vi "Lockin_time.vi"(8 "error in (no error)":errorcluster, 11 "Transport":refnum<class "Transport.lvclass">) -> (0 "error out":errorcluster, 3 "Transport out":refnum<class "Transport.lvclass">)   [LabVIEW 2019, in "Transport.lvclass"]
uses:
  Transport.lvclass
  Control Experiment/Control Experiment.lvclass
  <userlib>/LevyLab/Lockin-Multichannel/Instrument.Lockin/Instrument.Lockin.lvclass
  <userlib>/LevyLab/Lockin-Multichannel/Instrument.Lockin/Typedefs/Results Type--Enum.ctl
  <vilib>/PRIrvin/XY Utilities/xy_utilities.lvlib
  <vilib>/PRIrvin/XY Utilities/subVIs/Divide float (multiple).vi
  <vilib>/PRIrvin/XY Utilities/subVIs/Multiply float (multiple).vi
  8746f36a-7fba-47b8-9d0d-e5093f5f71bf.vi
  f6961605-28f7-45ab-8853-bc719731420b.vi
  <vilib>/PRIrvin/XY Utilities/subVIs/Get X and Y (single).vi
  <userlib>/LevyLab/Instrument Framework/Instrument Types/Cryostat/Typedefs/Magnet Mode--Enum.ctl
  <userlib>/LevyLab/Instrument Framework/Instrument Types/Cryostat/Instrument.Cryostat.lvclass
  <vilib>/Utility/Data Type/NI_Data Type.lvlib
  C:/Program Files/National Instruments/LabVIEW 2019/vi.lib/JKI/JKI SMO/SMO/SMO.lvclass
  <userlib>/LevyLab/Instrument Framework/Instrument Types/Lockin/Instrument.LockinAPI.lvclass
  <userlib>/LevyLab/Instrument Framework/Instrument Types/Amplifier/Instrument.Amplifier.lvclass
  <userlib>/LevyLab/Instrument Framework/Instrument Types/CBridge/Instrument.CBridge.lvclass
  <userlib>/LevyLab/Instrument Framework/Instrument Types/Delay Line/Instrument.DelayLine.lvclass
  <userlib>/LevyLab/Instrument Framework/Instrument Types/Strain/Instrument.Strain.lvclass
  <userlib>/LevyLab/Instrument Framework/Instrument Types/VNA/Instrument.VNA.lvclass
  <userlib>/LevyLab/Instrument Framework/Instrument Types/VSource/Instrument.VSource.lvclass
  Control Experiment/Typedefs/Instrument Types--enum.ctl
  <userlib>/LevyLab/Instrument Framework/Instrument/Instrument.lvclass
  Attributes/Instrument Attributes.lvlib
  <vilib>/PRIrvin/XY Utilities/subVIs/Get X and Y (multiple).vi
  <userlib>/LevyLab/Debug/Debug.lvlib
  28257cb1-27ee-4ed9-8846-d02f057abbea.vi
  C:/Program Files/National Instruments/LabVIEW 2019/user.lib/LevyLab/Instrument Framework/Instrument Types/Lockin/Instrument.LockinAPI.lvclass
  <userlib>/LevyLab/Instrument Framework/Instrument Types/Cryostat/Typedefs/Magnet Axis--Enum.ctl
panel:
  in  "Stop":bool
  in  "Tab Control":T1(tab)
  in  "Hold?":bool
  out "Instrument Status":string
  out "Mean":dbl[](array[numeric]) format="%#_6p"
  in  "refresh (ms)":u32=1000
  out "Experiment Description":string="this is the experiment description"
  out "Experiment Folder":string="1 -  Folder Name"
  out "X Channels":dbl[](array[numeric]) format="%#_6p"
  out "Y Channels":dbl[](array[numeric]) format="%#_6p"
  out "State History":string
  in  "T_hold (K)":dbl=1000.0
  out "Y":cluster{"Wavenumber":dbl[], "Data":dbl[]}[](graph)
  out "X":cluster{"Y":dbl[], "Y":dbl[]}[](graph)
  out "Mean":cluster{"Wavenumber":dbl[], "Data":dbl[]}[](graph)
  out "X (2)":cluster{"Y":dbl[], "Y":dbl[]}[](graph)
  in  "Units":enum16{"ohms & siemens", "h/e2 & e2/h"}(ring)
  out "G vs time":cluster{"Wavenumber":dbl[], "Data":dbl[]}[](graph)
  out "R vs time":cluster{"Wavenumber":dbl[], "Data":dbl[]}[](graph)
  in  "Electrodes":T2(array[cluster])
  out "T vs time":cluster{"X-array":dbl[], "Y-array":dbl[]}[](graph)
  out "R vs T":cluster{"Wavenumber":dbl[], "Data":dbl[]}[](graph)
  out "B vs time":cluster{"X-array":dbl[], "Y-array":dbl[]}[](graph)
  out "R vs B":cluster{"Wavenumber":dbl[], "Data":dbl[]}[](graph)
  in  "Axis":T3
  out "Angle vs time":cluster{"X-array":dbl[], "Y-array":dbl[]}[](graph)
  out "R vs Angle":cluster{"Wavenumber":dbl[], "Data":dbl[]}[](graph)
  # "Measurements"
  # "Configuration"
  # "Status"
  # "Metadata*"
  # "VI Description"
  # "Record the lockin outputs, along with the other configured instruments, as a function of time. On each refresh interval it reads every instrument and records one point. It runs until stopped. The refresh time can be changed while the VI is running (setRefreshTime)."
  # "*Change these values in Transport Server"
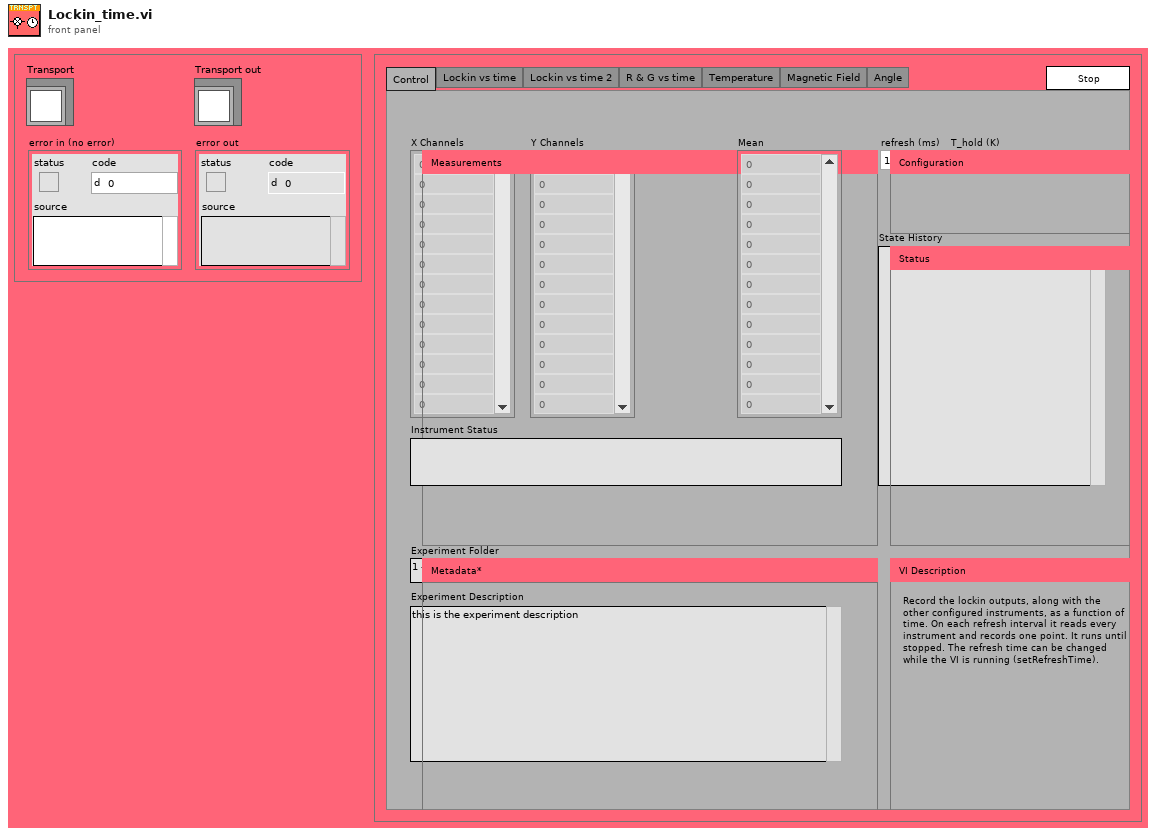
[diagram p1: front panel]
types:
  T1 = enum32{"Control", "Lockin vs time", "Lockin vs time 2", "R & G vs time", "Temperature", "Magnetic Field", "Angle"}
  T2 = cluster{"I+":i32, "I-":i32, "V+":i32, "V-":i32}[]
  T3 = typedef "Instrument.Cryostat.lvclass/Magnet Axis--Enum.ctl" = enum16{"X", "Y", "Z"}
  T4 = enum32{"Invalid", "Standard", "Closed", "Hidden", "Minimized", "Maximized"}
  T5 = enum32{"invalid app kind", "Development System", "Run Time System", "Student Edition", "Embedded LabVIEW", "Evaluation", "Custom"}
  T6 = typedef "Control Experiment.lvclass/Instrument Types--enum.ctl" = enum16{"DAQ", "Amplifier", "Temperature", "Magnet", "Rotator", "Level", "Capacitance", "Delay Line", "Strain Cell", "VNA", "Source"}
  T7 = typedef "Instrument.Cryostat.lvclass/Magnet Mode--Enum.ctl" = enum16{"Persistent", "Driven"}
  T8 = typedef "Instrument.Lockin.lvlib/Instrument.Lockin.lvclass/Results Type--Enum.ctl" = enum16{"X", "Y", "R", "Theta", "Mean"}
  T9 = typedef "Control Experiment.lvclass/Instrument Classes--cluster.ctl" = cluster{"DAQ":refnum<class "Instrument.LockinAPI.lvclass">, "Amplifier":refnum<class "Instrument.Amplifier.lvclass">, "Temperature":refnum<class "Instrument.Cryostat.lvclass">, "Magnet":refnum<class "Instrument.Cryostat.lvclass">, "Rotator":refnum<class "Instrument.Cryostat.lvclass">, "Level":refnum<class "Instrument.Cryostat.lvclass">, "Capacitance":refnum<class "Instrument.CBridge.lvclass">, "Delay Line":refnum<class "Instrument.DelayLine.lvclass">, "Strain Cell":refnum<class "Instrument.Strain.lvclass">, "VNA":refnum<class "Instrument.VNA.lvclass">, "Source":refnum<class "Instrument.VSource.lvclass">}
  T10 = cluster{"Core":cluster{"Current VI Reference":refnum<vi>, "Close Panel on Exit?":bool}, "Transport":refnum<class "Transport.lvclass">, "C.E.":refnum<class "Control Experiment.lvclass">, "Instruments":T9, "path":path, "time":dbl, "temperature":dbl, "magnet field":dbl, "magnet rate":dbl, "magnet hold":dbl, "magnet rate hold":dbl, "angle":dbl, "Lockin X":dbl[], "Lockin Y":dbl[], "Lockin Mean":dbl[], "Excitation":dbl[], "AO":dbl[], "AI":dbl[], "R2T":dbl[], "R4T":dbl[], "G2T":dbl[], "G4T":dbl[], "Execution:State":enum32{"Bad", "Idle", "Run top level", "Running"}}
  T11 = enum32{"Bad", "Idle", "Run top level", "Running"}
  T12 = cluster{"Current VI Reference":refnum<vi>, "Close Panel on Exit?":bool}
  T13 = cluster{"I-":i32, "I+":i32, "V1-":i32, "V1+":i32, "I2-":i32, "I2+":i32, "V2-":i32, "V2+":i32}
  T14 = typedef "LV-Data.lvclass/Dictionary--cluster.ctl" = cluster{"key":string, "value":variant}
  T15 = typedef "Instrument.Lockin.lvlib/Instrument.DAQ.lvclass/AO.Channel--Cluster--Array.ctl" = T16[]
  T16 = typedef "Instrument.Lockin.lvlib/Instrument.DAQ.lvclass/AO.Channel--Cluster.ctl" = cluster{"Enable?":bool, "Channel":i32, "Amplitude":dbl, "Offset":dbl, "Frequency":dbl, "Phase":dbl, "Function":T17, "Sweeping?":bool, "Limit AC":bool, "Limit DC?":bool, "Duty Cycle":bool}
  T17 = typedef "Instrument.Lockin.lvlib/Instrument.DAQ.lvclass/AO.Channel.Function--Enum.ctl" = enum16{"sine", "square", "triangle", "saw"}
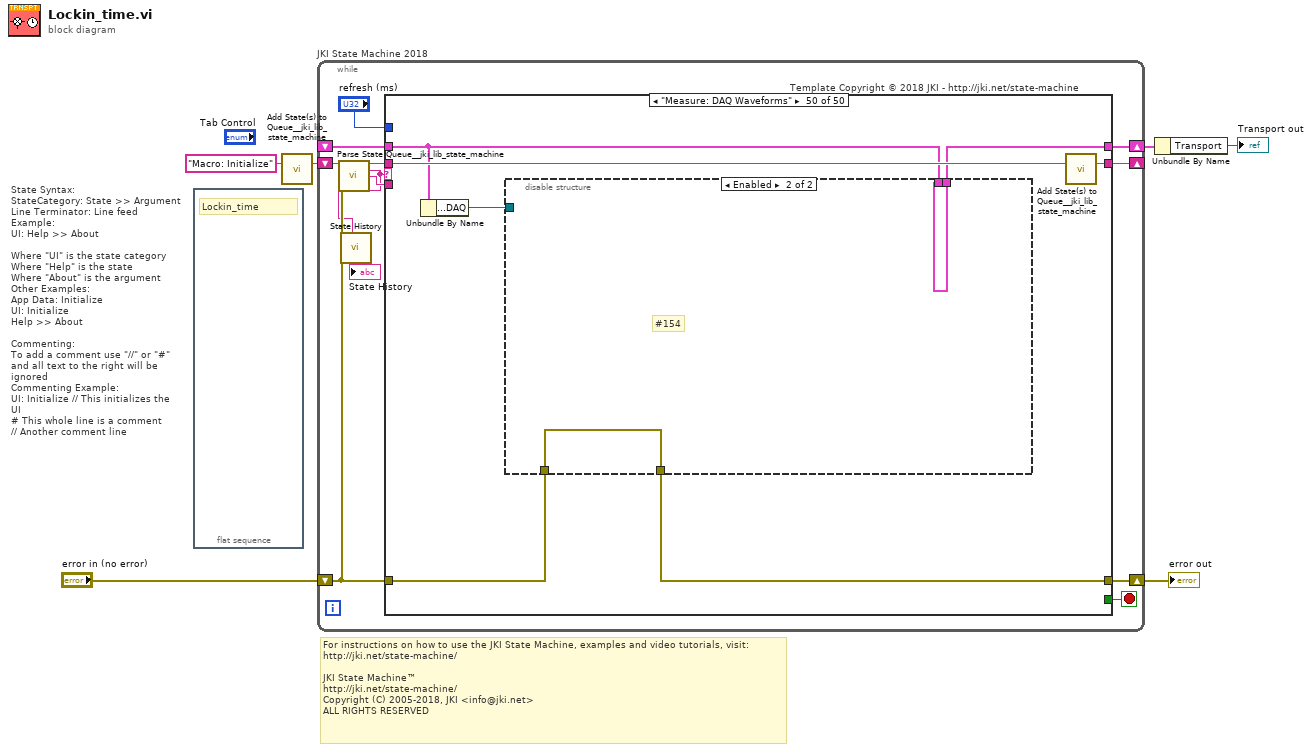
[diagram p0: block diagram]
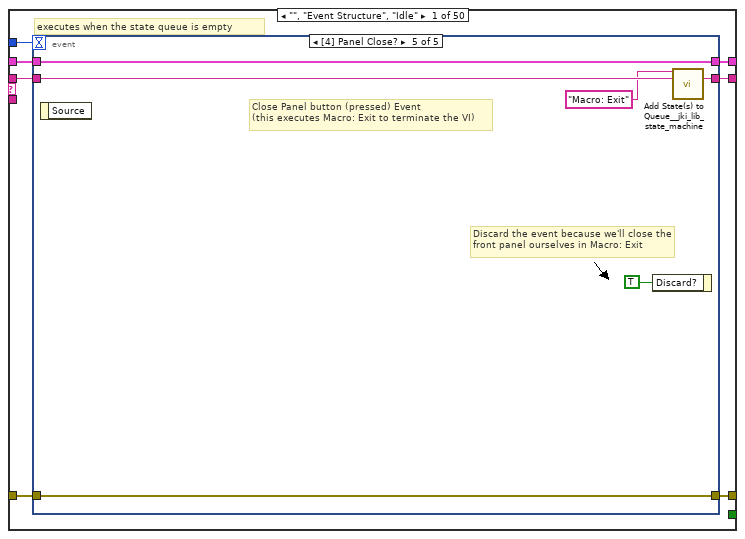
[diagram p2: hidden frame]
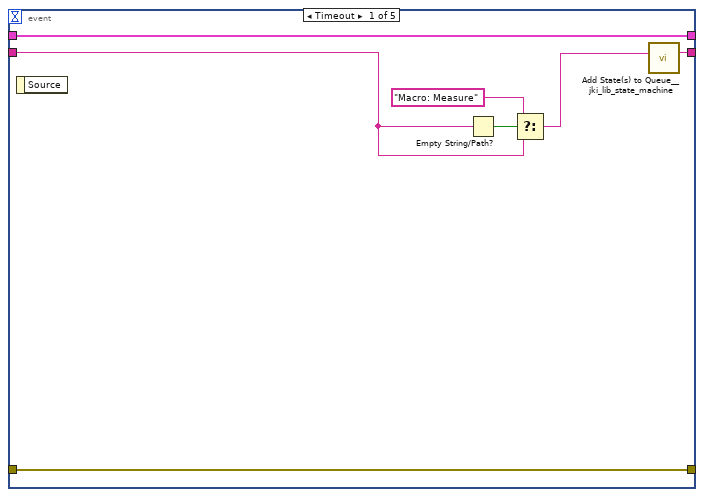
[diagram p3: hidden frame]
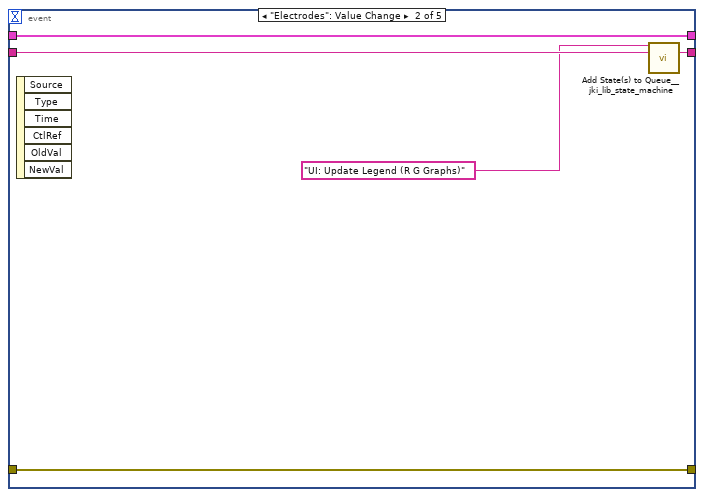
[diagram p4: hidden frame]
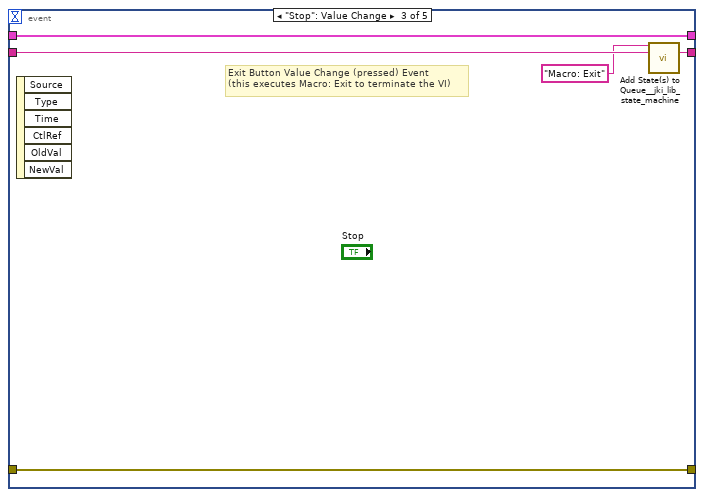
[diagram p5: hidden frame]
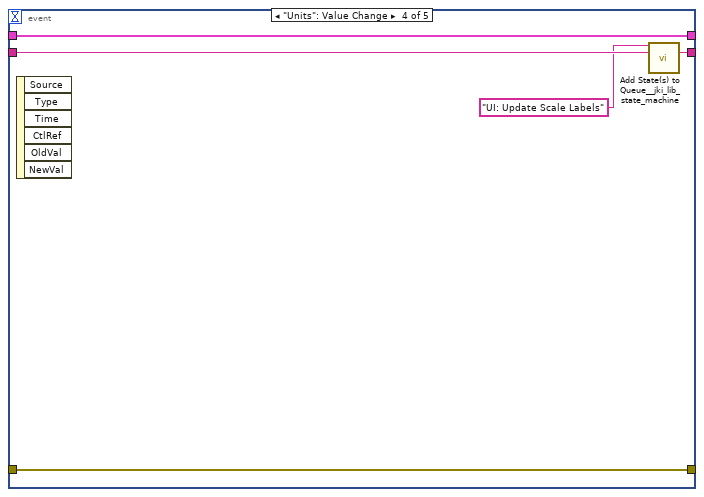
[diagram p6: hidden frame]
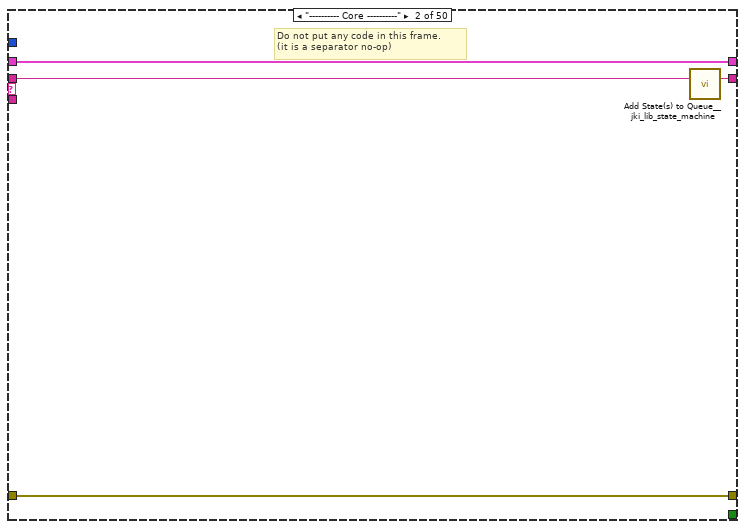
[diagram p7: hidden frame]
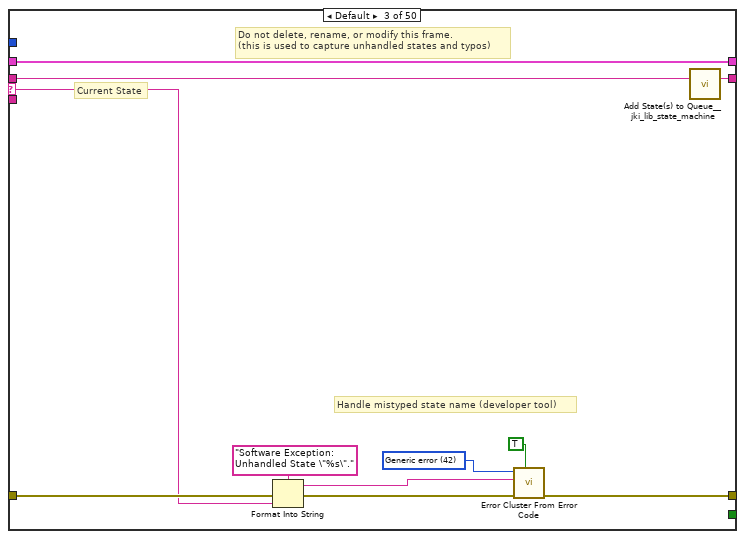
[diagram p8: hidden frame]
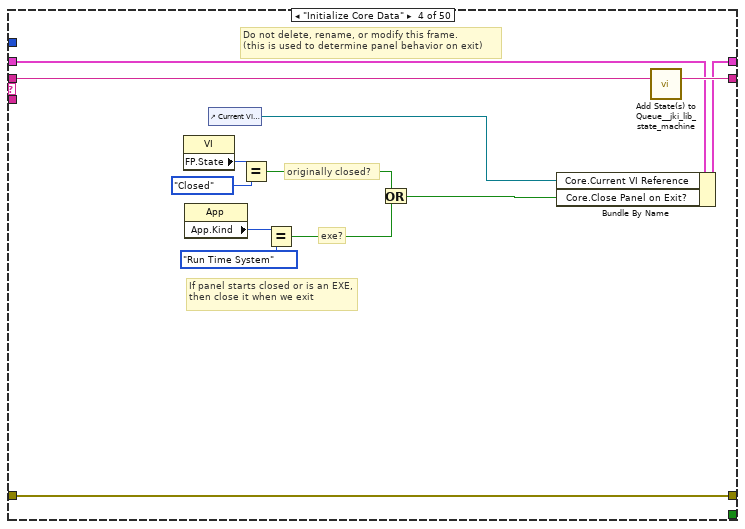
[diagram p9: hidden frame]
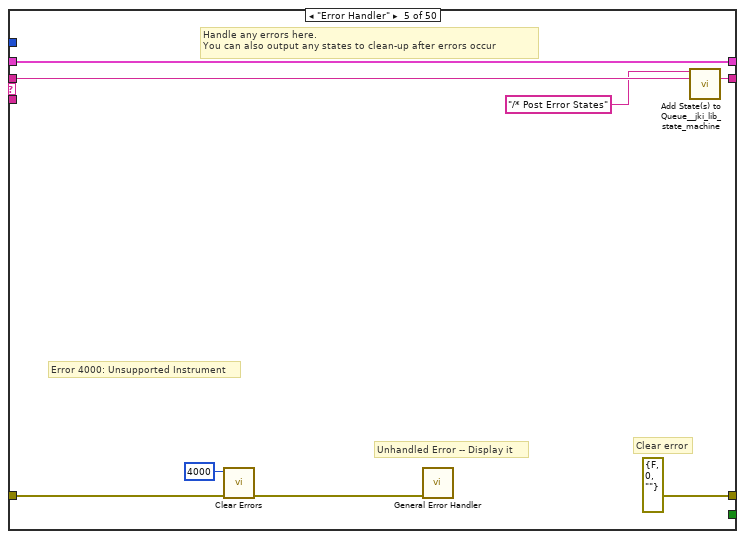
[diagram p10: hidden frame]
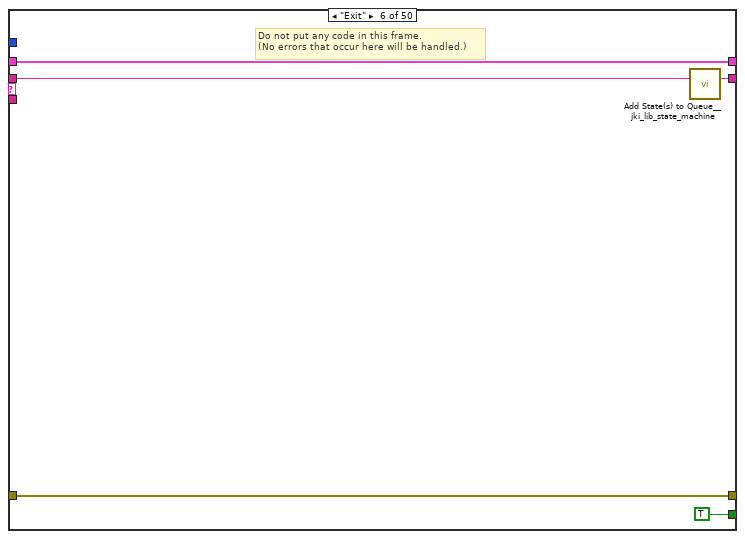
[diagram p11: hidden frame]
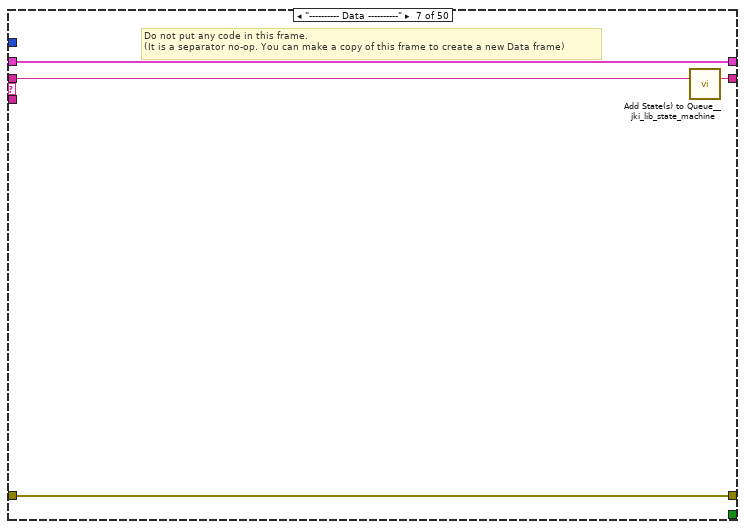
[diagram p12: hidden frame]
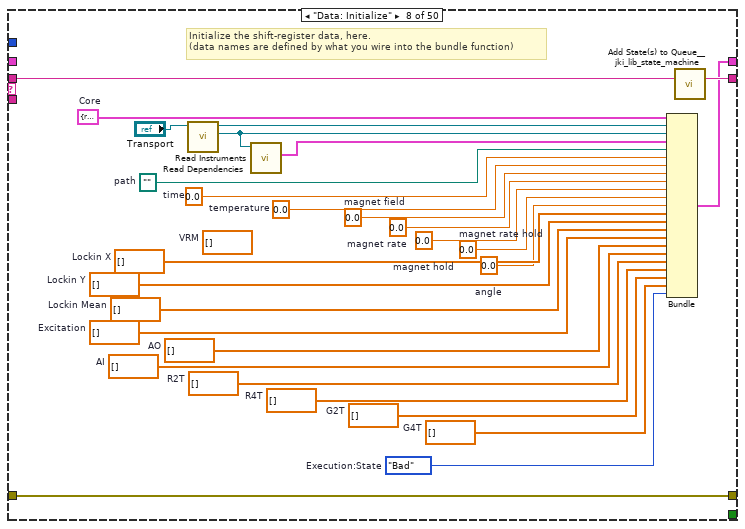
[diagram p13: hidden frame]
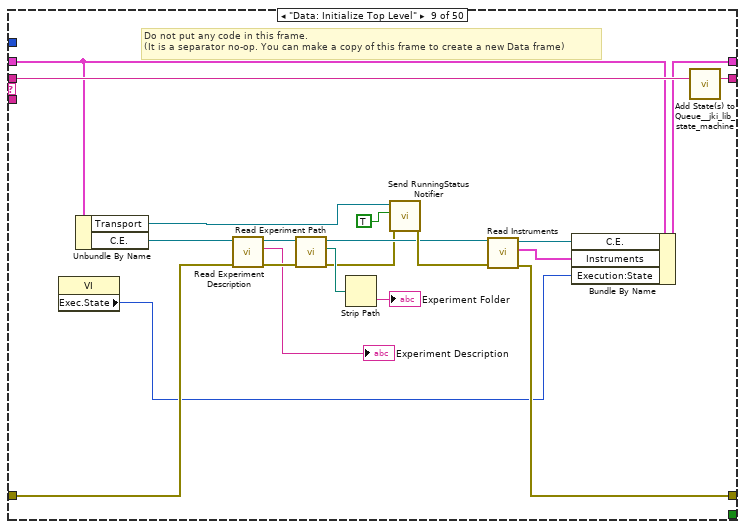
[diagram p14: hidden frame]
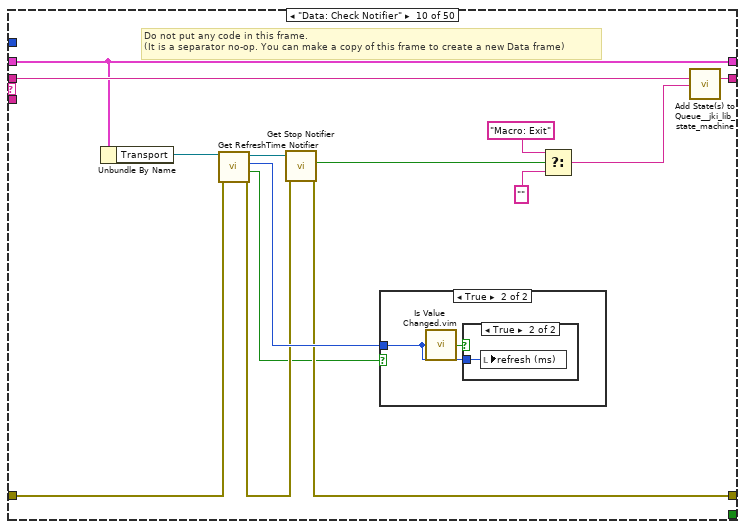
[diagram p15: hidden frame]
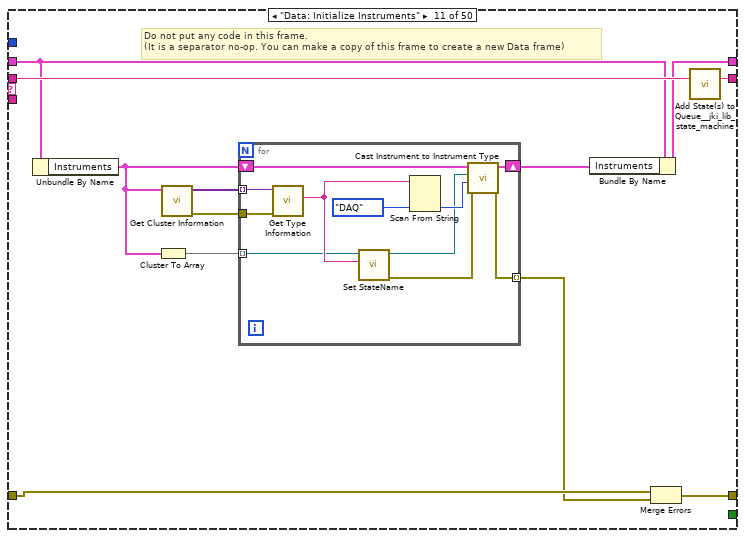
[diagram p18: hidden frame]
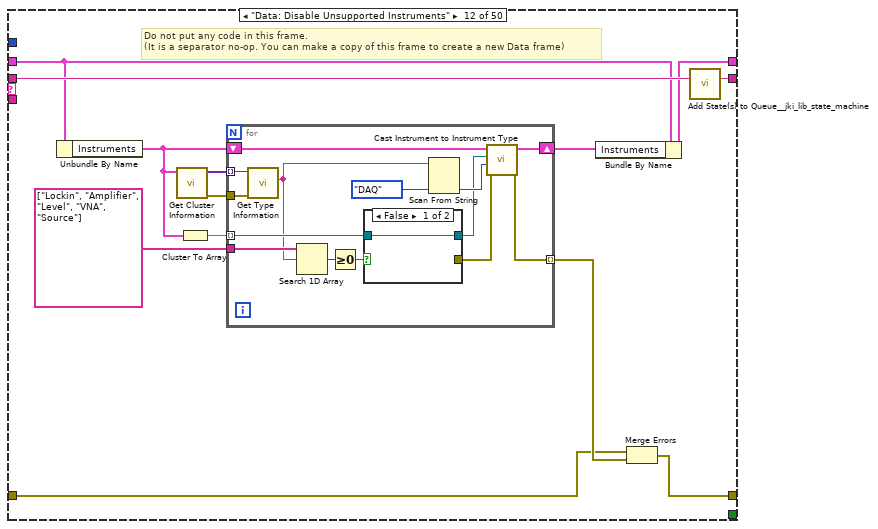
[diagram p19: hidden frame]
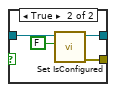
[diagram p20: hidden frame]
diagram:
  # "For instructions on how to use the JKI State Machine, examples and video tutorials, visit:\nhttp://jki.net/state-machine/\n\nJKI State Machine™\nhttp://jki.net/state-machine/\nCopyright (C) 2005-2018, JKI <info@jki.net>\nALL RIGHTS RESERVED"
  # "State Syntax:\nStateCategory: State >> Argument\nLine Terminator: Line feed\nExample:\nUI: Help >> About\n\nWhere \"UI\" is the state category\nWhere \"Help\" is the state\nWhere \"About\" is the argument\nOther Examples:\nApp Data: Initialize\nUI: Initialize\nHelp >> About\n\nCommenting:\nTo add a comment use \"//\" or \"#\" and all text to the right will be ignored\nCommenting Example:\nUI: Initialize // This initializes the UI\n# This whole line is a comment\n// Another comment line"
  n1 = flat-sequence {
    frame #0 {
      # "Lockin_time"
    }
  }
  n2 = call <vilib>:"Add State(s) to Queue__jki_lib_state_machine.vi"("State(s) in (\"\")"="Macro: Initialize") -> ("States Out"=w6:string)  [unwired: 14 in]
  n3 = while "JKI State Machine 2018" {
    shift-right: [w12] -> w2
    shift-left: _ -> [w11]
    shift-right: [w15] -> w3
    shift-left: "error in (no error)" -> [w10]
    shift-right: [w14] -> _
    shift-left: w6 -> [w16]
    stop <- w13 stop-if-true
    # "Template Copyright © 2018 JKI - http://jki.net/state-machine"
    n4 = call <vilib>:"Parse State Queue__jki_lib_state_machine.vi"("State Queue"=w16, "Error In (no error)"=w10) -> ("Remaining States"=w18:string, "Current State"=w8:string, "Arguments"=w17:string)  [unwired: 11 in]
    n5 = call <userlib>:"State History.vi"("Current State"=w8) -> ("History"=→"State History":string)  [unwired: 9 in, 1 out]
    n6 = case shown="\"Measure: DAQ Waveforms\"" w8 {
      selector: w8 -> [_ _ w58 _ _ _ _ _ _ _ _ _ _ _ _ _ _ _ _ _ _ _ _ _ _ _ _ _ _ _ _ _ _ _ _ _ _ _ _ _ _ _ _ _ _ _ _ _ _ _]
      tunnel: w18 -> [w25 w57 w62 w81 w89 w94 w98 w126 w146 w160 w175 w199 w230 w266 w278 w327 w348 w360 w366 w378 w413 w447 w466 w472 w483 w599 w630 w634 w639 w644 w649 w660 w673 w684 w688 w710 w725 w738 w749 w768 w802 w833 w845 w866 w899 w921 w943 w965 w999 w1009]
      tunnel: w17 -> [_ _ _ _ _ _ _ _ _ _ _ _ _ _ _ _ _ _ _ _ _ _ w452 w467 w477 w596 w624 _ _ _ _ _ _ _ _ w690 _ _ _ _ _ _ _ _ _ _ _ _ _ _]
      tunnel: w11 -> [w23 w54 w60 w74 w86 w92 w95 _ w142 w156 w172 w196 w227 w261 w275 w311 w345 w357 w363 w375 w410 w444 w463 w470 w479 w593 w627 w631 w636 w640 w646 w657 w670 w681 w685 w708 w716 w735 w742 w762 w795 w831 w843 w864 w889 w911 w933 w955 w996 w1006]
      tunnel: [w22 w55 w64 w78 errorcluster {"status"=FALSE, "code"=0, "source"=""} ("error out") w91 w96 w123 w137 w150 w171 w187 w226 w253 w274 w318 w343 w358 w362 w374 w405 w445 w464 w468 w480 w597 w628 w632 w637 w642 w647 w652 w671 w682 w686 w694 w718 w736 w740 w756 w790 w823 w839 w862 w887 w909 w931 w953 w980 w1004] -> w15
      tunnel: w10 -> [w21 w55 w63 w78 w82 w91 w96 w123 w141 w149 w165 w189 w225 w259 w273 w317 w341 w358 w364 w376 w411 w445 w464 w469 w481 w597 w628 w632 w637 w642 w647 w651 w671 w682 w686 w693 w720 w736 w739 w760 w793 w819 w836 w852 w891 w913 w935 w957 w973 w1003]
      tunnel: [w24 w56 w61 w80 w88 w93 w97 w125 w145 w159 w174 w198 w229 w265 w277 w326 w347 w359 w365 w377 w412 w446 w465 w471 w482 w598 w629 w633 w638 w643 w648 w659 w672 w683 w687 w709 w724 w737 w748 w767 w801 w832 w844 w865 w898 w920 w942 w964 w998 w1008] -> w14
      tunnel: [_ _ _ _ _ TRUE _ _ _ _ _ _ _ _ _ _ _ _ _ _ _ _ _ _ _ _ _ _ _ _ _ _ _ _ _ _ _ _ _ _ _ _ _ _ _ _ _ _ _ _] -> w13
      tunnel: [w20 w54 w60 w79 w86 w92 w95 w124 w143 w156 w173 w197 w228 w260 w276 w312 w344 w357 w363 w375 w410 w444 w463 w470 w479 w593 w627 w631 w636 w640 w646 w657 w670 w681 w685 w707 w717 w735 w741 w761 w794 w830 w842 w863 w890 w912 w934 w956 w997 w1007] -> w12
      tunnel: "refresh (ms)" -> [w19 _ _ _ _ _ _ _ _ _ _ _ _ _ _ _ _ _ _ _ _ _ _ _ _ _ _ _ _ _ _ _ _ _ _ _ _ _ _ _ _ _ _ _ _ _ _ _ _ _]
      frame "", "Event Structure", "Idle" {
        # "executes when the state queue is empty"
        n7 = event shown="[4] Panel Close?" {
          selector: _ -> [_ _ _ _ _]
          dyn-events: _ -> [_ _ _ _ _]
          timeout: w19 -> [_ _ _ _ _]
          tunnel: w25 -> [w28 w37 w42 w47 w53]
          tunnel: [w32 w36 w41 w46 w52] -> w24
          tunnel: w23 -> [w30 w34 w39 w44 w50]
          tunnel: [w31 w35 w40 w45 w51] -> w22
          tunnel: w21 -> [w31 w35 w40 w45 w51]
          tunnel: [w30 w34 w39 w44 w50] -> w20
          event Timeout {
            n8 = event-data() -> ()  [unwired: 1 in, 1 out]
            n9 = Empty String/Path?(string/path=w28) -> (empty?=w29:bool)
            n10 = Select(t="Macro: Measure" ("State(s) in Front (\"\")"), s=w29, f=w28) -> (s? t:f=w26:string)
            n11 = call <vilib>:"Add State(s) to Queue__jki_lib_state_machine.vi"("State(s) in (\"\")"=w26) -> ("States Out"=w32:string)  [unwired: 14 in]
          }
          event "Electrodes": Value Change {
            n12 = event-data() -> ()  [unwired: 1 in, 6 out]
            n13 = call <vilib>:"Add State(s) to Queue__jki_lib_state_machine.vi"("State(s) in Front (\"\")"="UI: Update Legend (R G Graphs)" ("State(s) in Front (\"\")"), "State(s) in (\"\")"=w37) -> ("States Out"=w36:string)  [unwired: 13 in]
          }
          event "Stop": Value Change {
            # "Exit Button Value Change (pressed) Event\n(this executes Macro: Exit to terminate the VI)"
            n14 = event-data() -> ()  [unwired: 1 in, 6 out]
            n15 = call <vilib>:"Add State(s) to Queue__jki_lib_state_machine.vi"("State(s) in Front (\"\")"="Macro: Exit", "State(s) in (\"\")"=w42) -> ("States Out"=w41:string)  [unwired: 13 in]
          }
          event "Units": Value Change {
            n16 = event-data() -> ()  [unwired: 1 in, 6 out]
            n17 = call <vilib>:"Add State(s) to Queue__jki_lib_state_machine.vi"("State(s) in Front (\"\")"="UI: Update Scale Labels", "State(s) in (\"\")"=w47) -> ("States Out"=w46:string)  [unwired: 13 in]
          }
          event Panel Close? {
            # "Discard the event because we'll close the front panel ourselves in Macro: Exit"
            # "Close Panel button (pressed) Event\n(this executes Macro: Exit to terminate the VI)"
            n18 = event-data() -> ()  [unwired: 1 in, 1 out]
            n19 = event-data("Discard?"=TRUE) -> ()  [unwired: 1 in, 1 out]
            n20 = call <vilib>:"Add State(s) to Queue__jki_lib_state_machine.vi"("State(s) in Front (\"\")"="Macro: Exit", "State(s) in (\"\")"=w53) -> ("States Out"=w52:string)  [unwired: 13 in]
          }
        }
      }
      frame "---------- Core ----------" {
        # "Do not put any code in this frame.\n(it is a separator no-op)"
        n21 = call <vilib>:"Add State(s) to Queue__jki_lib_state_machine.vi"("State(s) in (\"\")"=w57) -> ("States Out"=w56:string)  [unwired: 14 in]
      }
      frame Default {
        w67 = 42 items=["No error", "Argument error", "Memory is full", "Out of zone", "End of file", "File already open", "Generic file I/O error", "File not found", "File permission error", "Disk is full", "Duplicate path", "Too many files open", "System feature not enabled", "Resource file not found", "Cannot add resource", "Resource not found", "Image not found", "Image memory error", "Pen does not exist", "Config type invalid", "Config token not found", "Config parse error", "Config memory error", "Bad external code format", "Bad external code offset", "External code not present", "Null window", "Destroy window error", "Null menu", "Print aborted", "Bad print record", "Print driver error", "Windows error during printing", "Memory error during printing", "Print dialog error", "Generic print error", "Invalid device refnum", "Device not found", "Device parameter error", "Device unit error", "Cannot open device", "Device call aborted", "Generic error", "Cancelled by user", "Object ID too low", "Object ID too high", "Object not in heap", "Unknown heap", "Unknown object (invalid DefProc)", "Unknown object (DefProc not in table)", "Message out of range", "Invalid (null) method", "Unknown message", "Manager call not supported", "Bad address", "Network operation in progress", "Network operation timed out", "Connection is busy", "Network attribute not supported", "Network error", "Address in use", "System out of memory", "Connection aborted", "Connection refused", "Not connected", "Already connected", "Connection closed", "Initialization error (interapplication manager)", "Bad occurrence", "Wait on unbound occurrence handler", "Occurrence queue overflow", "Datalog type conflict", "Unused", "Unrecognized type (interapplication manager)", "Memory corrupt", "Failed to make temporary DLL", "Old CIN version", "Drag socket not found", "Failed to load drop-object", "Failed to register OLE object", "Failed to release OLE object", "Format specifier type mismatch", "Unknown format specifier", "Too few format specifiers", "Too many format specifiers", "Scan failed", "Newer CIN version", "Error converting to variant", "Runtime menu error", "Password tampered", "Variant attribute not found", "Incompatible variant data type", "Event data is not available", "Event Store is not present", "Occurrence is not found", "Event Queue is not created", "Event info is not available", "Refnum passed is NULL", "Error retrieving Class GUID", "Error retrieving CoClass GUID", "Error retrieving TypeLib GUID.", "Bad built application magic bytes.", "Specific driver is different from the specific driver associated with the Logical Name.", "There is no session opened to the class driver.", "Max Error", "MAX - Error with config objects", "MAX - Error loading configuration", "MAX - Group not supported"]
        # "Current State"
        # "Do not delete, rename, or modify this frame.\n(this is used to capture unhandled states and typos)"
        # "Handle mistyped state name (developer tool)"
        n22 = Format Into String(format string="Software Exception: Unhandled State \"%s\"." ("message"), error in=w63, w58) -> (resulting string=w66:string, error out=w65:errorcluster)  [unwired: 1 in]
        n23 = call <vilib>:"Error Cluster From Error Code.vi"("show call chain? (False)"=TRUE, "error in (no error)"=w65, "error message (\"\")"=w66, "error code (0)"=w67) -> ("error out"=w64:errorcluster)  [unwired: 5 in]
        n24 = call <vilib>:"Add State(s) to Queue__jki_lib_state_machine.vi"("State(s) in (\"\")"=w62) -> ("States Out"=w61:string)  [unwired: 14 in]
      }
      frame "Initialize Core Data" {
        # "Do not delete, rename, or modify this frame.\n(this is used to determine panel behavior on exit)"
        # "originally closed?"
        # "exe?"
        # "If panel starts closed or is an EXE, then close it when we exit"
        n25 = property class="VI"() -> ("FP.State"=w71:T4)  [unwired: 2 in, 2 out]
        n26 = property class="App"() -> ("App.Kind"=w77:T5)  [unwired: 2 in, 2 out]
        n27 = control-ref of="Current VI Reference"() -> (w72:refnum<vi>)
        n28 = Equal?(x=w71, y=T4."Closed" ("Front Panel Window:State")) -> (x = y?=w69:bool)
        n29 = Equal?(x=w77, y=T5."Run Time System" ("Application:Kind")) -> (x = y?=w75:bool)
        n30 = Or(x=w69, y=w75) -> (x .or. y?=w73:bool)
        n31 = Bundle By Name(cluster=w74, "Core.Current VI Reference"=w72, "Core.Close Panel on Exit?"=w73) -> (w79:T10)
        n32 = call <vilib>:"Add State(s) to Queue__jki_lib_state_machine.vi"("State(s) in (\"\")"=w81) -> ("States Out"=w80:string)  [unwired: 14 in]
      }
      frame "Error Handler" {
        # "Error 4000: Unsupported Instrument"
        # "Unhandled Error -- Display it"
        # "Handle any errors here.\nYou can also output any states to clean-up after errors occur"
        # "Clear error"
        n33 = call <vilib>:"Clear Errors.vi"("error in (no error)"=w82, "specific error code to clear (0: all)"=4000) -> ("error out"=w83:errorcluster)  [unwired: 4 in, 1 out]
        n34 = call <vilib>:"General Error Handler.vi"("error in (no error)"=w83) -> ()  [unwired: 10 in, 5 out]
        n35 = call <vilib>:"Add State(s) to Queue__jki_lib_state_machine.vi"("State(s) in Front (\"\")"="/* Post Error States", "State(s) in (\"\")"=w89) -> ("States Out"=w88:string)  [unwired: 13 in]
      }
      frame "Exit" {
        # "Do not put any code in this frame.\n(No errors that occur here will be handled.)"
        n36 = call <vilib>:"Add State(s) to Queue__jki_lib_state_machine.vi"("State(s) in (\"\")"=w94) -> ("States Out"=w93:string)  [unwired: 14 in]
      }
      frame "---------- Data ----------" {
        # "Do not put any code in this frame.\n(It is a separator no-op. You can make a copy of this frame to create a new Data frame)"
        n37 = call <vilib>:"Add State(s) to Queue__jki_lib_state_machine.vi"("State(s) in (\"\")"=w98) -> ("States Out"=w97:string)  [unwired: 14 in]
      }
      frame "Data: Initialize" {
        w99 = 0.0  # angle
        w101 = 0.0  # magnet rate
        w102 = 0.0  # magnet rate hold
        w103 = 0.0  # magnet hold
        (unwired) dbl[] []  # VRM
        w106 = dbl[] []  # Excitation
        w109 = dbl[] []  # Lockin Mean
        w108 = dbl[] []  # AI
        w107 = dbl[] []  # AO
        w111 = T11."Bad"  # Execution:State
        w112 = dbl[] []  # G4T
        w113 = dbl[] []  # G2T
        w114 = dbl[] []  # R4T
        w115 = dbl[] []  # R2T
        w116 = dbl[] []  # Lockin Y
        w117 = dbl[] []  # Lockin X
        w118 = 0.0  # magnet field
        w119 = 0.0  # temperature
        w120 = 0.0  # time
        w121 = path ""  # path
        w122 = T12 {"Current VI Reference"=refnum, "Close Panel on Exit?"=FALSE}  # Core
        # "Initialize the shift-register data, here.\n(data names are defined by what you wire into the bundle function)"
        n38 = call "Read Dependencies.vi"("Transport"="Transport") -> ("C.E."=w105:refnum<class "Control Experiment.lvclass">, "Transport"=w100:refnum<class "Transport.lvclass">)  [unwired: 8 in, 1 out]
        n39 = call "Read Instruments.vi"("Control Experiment in"=w105) -> ("Instruments"=w104:T9)  [unwired: 8 in, 2 out]
        n40 = Bundle("Core"=w122, "Transport"=w100, "C.E."=w105, "Instruments"=w104, "path"=w121, "time"=w120, "temperature"=w119, "magnet field"=w118, "magnet rate"=w101, "magnet hold"=w103, "magnet rate hold"=w102, "angle"=w99, "Lockin X"=w117, "Lockin Y"=w116, "Lockin Mean"=w109, "Excitation"=w106, "AO"=w107, "AI"=w108, "R2T"=w115, "R4T"=w114, "G2T"=w113, "G4T"=w112, "Execution:State"=w111) -> (w124:T10)  [unwired: 1 in]
        n41 = call <vilib>:"Add State(s) to Queue__jki_lib_state_machine.vi"("State(s) in (\"\")"=w126) -> ("States Out"=w125:string)  [unwired: 14 in]
      }
      frame "Data: Initialize Top Level" {
        # "Do not put any code in this frame.\n(It is a separator no-op. You can make a copy of this frame to create a new Data frame)"
        n42 = property class="VI"() -> ("Exec.State"=w136:T11)  [unwired: 2 in, 2 out]
        n43 = Unbundle By Name(w142) -> ("Transport"=w134:refnum<class "Transport.lvclass">, "C.E."=w144:refnum<class "Control Experiment.lvclass">)
        n44 = call "Read Experiment Description.vi"("error in (no error)"=w141, "Control Experiment in"=w144) -> ("error out"=w132:errorcluster, "Experiment Description"=→"Experiment Description":string, "Control Experiment out"=w131:refnum<class "Control Experiment.lvclass">)  [unwired: 7 in]
        n45 = call "Read Experiment Path.vi"("error in (no error)"=w132, "Control Experiment in"=w131) -> ("error out"=w130:errorcluster, "Experiment Path"=w133:path, "Control Experiment out"=w139:refnum<class "Control Experiment.lvclass">)  [unwired: 7 in]
        n46 = Strip Path(path=w133) -> (name=→"Experiment Folder":string)  [unwired: 1 out]
        n47 = call "Send RunningStatus Notifier.vi"("error in (no error)"=w130, "Running?"=TRUE, "Transport in"=w134) -> ("error out"=w140:errorcluster)  [unwired: 7 in, 1 out]
        n48 = call "Read Instruments.vi"("error in (no error)"=w140, "Control Experiment in"=w139) -> ("error out"=w137:errorcluster, "Instruments"=w135:T9, "Control Experiment out"=w138:refnum<class "Control Experiment.lvclass">)  [unwired: 7 in]
        n49 = Bundle By Name(cluster=w142, "C.E."=w138, "Instruments"=w135, "Execution:State"=w136) -> (w143:T10)
        n50 = call <vilib>:"Add State(s) to Queue__jki_lib_state_machine.vi"("State(s) in (\"\")"=w146) -> ("States Out"=w145:string)  [unwired: 14 in]
      }
      frame "Data: Check Notifier" {
        # "Do not put any code in this frame.\n(It is a separator no-op. You can make a copy of this frame to create a new Data frame)"
        n51 = Unbundle By Name(w156) -> ("Transport"=w153:refnum<class "Transport.lvclass">)
        n52 = call "Get RefreshTime Notifier.vi"("error in (no error)"=w149, "Transport in"=w153) -> ("error out"=w148:errorcluster, "valid?"=w147:bool, "RefreshTime (ms)"=w151:u32, "Transport out"=w152:refnum<class "Transport.lvclass">)  [unwired: 6 in]
        n53 = call "Get Stop Notifier.vi"("error in (no error)"=w148, "Transport in"=w152) -> ("error out"=w150:errorcluster, "Stop?"=w154:bool)  [unwired: 7 in, 1 out]
        n54 = case shown="True" w147 {
          tunnel: w151 -> [_ w161]
          frame False {
          }
          frame True {
            n55 = call "Is Value Changed.vim"("value"=w161) -> ("changed or first call?"=w162:bool)
            n56 = case shown="True" w162 {
              tunnel: w161 -> [_ w163]
              frame False {
              }
              frame True {
                n57 = local write "refresh (ms)"(w163) -> ()
              }
            }
          }
        }
        n58 = Select(t="Macro: Exit", s=w154, f="") -> (s? t:f=w155:string)
        n59 = call <vilib>:"Add State(s) to Queue__jki_lib_state_machine.vi"("State(s) in (\"\")"=w160, "State(s) at Back (\"\")"=w155) -> ("States Out"=w159:string)  [unwired: 13 in]
      }
      frame "Data: Initialize Instruments" {
        # "Do not put any code in this frame.\n(It is a separator no-op. You can make a copy of this frame to create a new Data frame)"
        n60 = Unbundle By Name(w172) -> ("Instruments"=w166:T9)
        n61 = Cluster To Array(cluster=w166) -> (array=w170:refnum<class "Instrument.lvclass">[])
        n62 = call <vilib>:"Get Cluster Information.vi"("variant"=w166) -> ("error out"=w168:errorcluster, "cluster elements"=w169:variant[])  [unwired: 9 in]
        n63 = for {
          tunnel: w170 -> [w176] mode=indexing
          tunnel: [w184] -> w164 mode=indexing
          shift-right: [w185] -> w167
          shift-left: w166 -> [w186]
          tunnel: w169 -> [w181] mode=indexing
          tunnel: w168 -> [w180]
          n64 = call <vilib>:"Get Type Information.vi"("error in (no error)"=w180, "variant"=w181) -> ("name"=w177:string)  [unwired: 5 in, 4 out]
          n65 = call "Set StateName.vi"("StateName"=w177, "SMO"=w176) -> ("error out"=w178:errorcluster, "SMO out"=w179:refnum<class "Instrument.lvclass">)  [unwired: 8 in]
          n66 = Scan From String(input string=w177, default 1=Instrument_Types--enum."DAQ" ("Type")) -> (output 1=w182:T6)  [unwired: 3 in, 3 out]
          n67 = call "Cast Instrument to Instrument Type.vi"("error in (no error)"=w178, "Type"=w182, "Instrument in"=w179, "Instrument Classes"=w186) -> ("error out"=w184:errorcluster, "Instrument Classes out"=w185:T9)  [unwired: 5 in, 1 out]
        }
        n68 = Bundle By Name(cluster=w172, "Instruments"=w167) -> (w173:T10)
        n69 = Merge Errors(w165, w164) -> (w171:errorcluster)
        n70 = call <vilib>:"Add State(s) to Queue__jki_lib_state_machine.vi"("State(s) in (\"\")"=w175) -> ("States Out"=w174:string)  [unwired: 14 in]
      }
      frame "Data: Disable Unsupported Instruments" {
        # "Do not put any code in this frame.\n(It is a separator no-op. You can make a copy of this frame to create a new Data frame)"
        n71 = Unbundle By Name(w196) -> ("Instruments"=w192:T9)
        n72 = call <vilib>:"Get Cluster Information.vi"("variant"=w192) -> ("error out"=w193:errorcluster, "cluster elements"=w194:variant[])  [unwired: 9 in]
        n73 = Cluster To Array(cluster=w192) -> (array=w195:refnum<class "Instrument.lvclass">[])
        n74 = for {
          tunnel: w195 -> [w206] mode=indexing
          tunnel: [w211] -> w190 mode=indexing
          shift-right: [w212] -> w191
          shift-left: w192 -> [w213]
          tunnel: w194 -> [w208] mode=indexing
          tunnel: w193 -> [w207]
          tunnel: string[] ["Lockin", "Amplifier", "Level", "VNA", "Source"] ("element") -> [w203]
          n75 = call <vilib>:"Get Type Information.vi"("error in (no error)"=w207, "variant"=w208) -> ("name"=w202:string)  [unwired: 5 in, 4 out]
          n76 = Search 1D Array(1D array=w203, element=w202) -> (index of element=w200:i32)  [unwired: 1 in]
          n77 = Greater Or Equal To 0?(x=w200) -> (x >= 0?=w201:bool)
          n78 = case shown="False" w201 {
            tunnel: w206 -> [w214 w218]
            tunnel: [w214 w217] -> w205
            tunnel: [_ w216] -> w204
            frame False {
            }
            frame True {
              n79 = call "Set IsConfigured.vi"("IsConfigured?"=FALSE, "SMO"=w218) -> ("error out"=w216:errorcluster, "SMO out"=w217:refnum<class "Instrument.lvclass">)  [unwired: 8 in]
            }
          }
          n80 = Scan From String(input string=w202, default 1=Instrument_Types--enum."DAQ" ("Type")) -> (output 1=w209:T6)  [unwired: 3 in, 3 out]
          n81 = call "Cast Instrument to Instrument Type.vi"("error in (no error)"=w204, "Type"=w209, "Instrument in"=w205, "Instrument Classes"=w213) -> ("error out"=w211:errorcluster, "Instrument Classes out"=w212:T9)  [unwired: 5 in, 1 out]
        }
        n82 = Bundle By Name(cluster=w196, "Instruments"=w191) -> (w197:T10)
        n83 = Merge Errors(w189, w190) -> (w187:errorcluster)
        n84 = call <vilib>:"Add State(s) to Queue__jki_lib_state_machine.vi"("State(s) in (\"\")"=w199) -> ("States Out"=w198:string)  [unwired: 14 in]
      }
      frame "Data: Open Instruments" {
        # "Do not put any code in this frame.\n(It is a separator no-op. You can make a copy of this frame to create a new Data frame)"
        n85 = Unbundle By Name(w227) -> ("Instruments"=w221:T9)
        n86 = call <vilib>:"Get Cluster Information.vi"("variant"=w221) -> ("error out"=w222:errorcluster, "cluster elements"=w223:variant[])  [unwired: 9 in]
        n87 = Cluster To Array(cluster=w221) -> (array=w224:refnum<class "Instrument.lvclass">[])
        n88 = for {
          tunnel: w224 -> [w231] mode=indexing
          tunnel: [w241] -> w219 mode=indexing
          shift-right: [w243] -> w220
          shift-left: w221 -> [w244]
          tunnel: w223 -> [w238] mode=indexing
          tunnel: w222 -> [w237]
          n89 = call <vilib>:"Get Type Information.vi"("error in (no error)"=w237, "variant"=w238) -> ("name"=w232:string)  [unwired: 5 in, 4 out]
          n90 = call "Get IsConfigured.vi"("SMO"=w231) -> ("error out"=w233:errorcluster, "IsConfigured?"=w234:bool, "SMO out"=w235:refnum<class "Instrument.lvclass">)  [unwired: 8 in]
          n91 = case shown="True" w234 {
            tunnel: [w245 w250] -> w242
            tunnel: w235 -> [w246 w249]
            tunnel: [w246 w248] -> w236
            tunnel: w233 -> [w245 w247]
            frame False {
            }
            frame True {
              n92 = call-dynamic "Open.vi"("error in (no error)"=w247, "Instrument in"=w249) -> ("error out"=w250:errorcluster, "Instrument out"=w248:refnum<class "Instrument.lvclass">)  [unwired: 8 in]
            }
          }
          n93 = Scan From String(input string=w232, default 1=Instrument_Types--enum."DAQ" ("Type")) -> (output 1=w239:T6)  [unwired: 3 in, 3 out]
          n94 = call "Cast Instrument to Instrument Type.vi"("error in (no error)"=w242, "Type"=w239, "Instrument in"=w236, "Instrument Classes"=w244) -> ("error out"=w241:errorcluster, "Instrument Classes out"=w243:T9)  [unwired: 5 in, 1 out]
        }
        n95 = Bundle By Name(cluster=w227, "Instruments"=w220) -> (w228:T10)
        n96 = Merge Errors(w225, w219) -> (w226:errorcluster)
        n97 = call <vilib>:"Add State(s) to Queue__jki_lib_state_machine.vi"("State(s) in (\"\")"=w230) -> ("States Out"=w229:string)  [unwired: 14 in]
      }
      frame "Data: Configure Magnet Type" {
        # "show/hide\naxis control"
        # "Do not put any code in this frame.\n(It is a separator no-op. You can make a copy of this frame to create a new Data frame)"
        n98 = Unbundle By Name(w261) -> ("Instruments.Magnet"=w258:refnum<class "Instrument.Cryostat.lvclass">)
        n99 = call <vilib>:"Get LV Class Name.vi"("error in (no error)"=w259, "object"=w258) -> ("error out"=w254:errorcluster, "class name"=w264:string)  [unwired: 8 in]
        n100 = Match Pattern(string=w264, regular expression="VRM") -> (offset past match=w262:i32)  [unwired: 1 in, 3 out]
        n101 = Greater Or Equal To 0?(x=w262) -> (x >= 0?=w251:bool)
        n102 = Select(t="Vector Magnet" ("new element/subarray"), s=w251, f="Magnet" ("element")) -> (s? t:f=w252:string)
        n103 = call "Set StateName.vi"("error in (no error)"=w254, "StateName"=w252, "SMO"=w258) -> ("error out"=w253:errorcluster, "SMO out"=w257:refnum<class "Instrument.Cryostat.lvclass">)  [unwired: 7 in]
        n104 = Bundle By Name(cluster=w261, "Instruments.Magnet"=w257) -> (w260:T10)
        n105 = property on="Axis" class="Enum (strict)"("Visible"=w251) -> ()  [unwired: 2 in, 2 out]
        n106 = call <vilib>:"Add State(s) to Queue__jki_lib_state_machine.vi"("State(s) in (\"\")"=w266) -> ("States Out"=w265:string)  [unwired: 14 in]
      }
      frame "Data: Close Instruments" {
        # "Data: Close Instruments\n(Close Instruments that are explicitly opened by this VI)"
        n107 = Unbundle By Name(w275) -> ("Instruments"=w269:T9)
        n108 = call <vilib>:"Get Cluster Information.vi"("variant"=w269) -> ("error out"=w270:errorcluster, "cluster elements"=w271:variant[])  [unwired: 9 in]
        n109 = Cluster To Array(cluster=w269) -> (array=w272:refnum<class "Instrument.lvclass">[])
        n110 = for {
          tunnel: w272 -> [w280] mode=indexing
          tunnel: [w288] -> w267 mode=indexing
          shift-right: [w291] -> w268
          shift-left: w269 -> [w292]
          tunnel: w271 -> [w285] mode=indexing
          tunnel: w270 -> [w284]
          n111 = call <vilib>:"Get Type Information.vi"("error in (no error)"=w284, "variant"=w285) -> ("name"=w283:string)  [unwired: 5 in, 4 out]
          n112 = call "Get IsConfigured.vi"("SMO"=w280) -> ("error out"=w279:errorcluster, "IsConfigured?"=w282:bool, "SMO out"=w281:refnum<class "Instrument.lvclass">)  [unwired: 8 in]
          n113 = case shown="True" w282 {
            tunnel: [w293 w298] -> w289
            tunnel: w281 -> [w294 w297]
            tunnel: [w294 w296] -> w290
            tunnel: w279 -> [w293 w295]
            frame False {
            }
            frame True {
              n114 = call-dynamic "Close.vi"("error in (no error)"=w295, "Instrument in"=w297) -> ("error out"=w298:errorcluster, "Instrument out"=w296:refnum<class "Instrument.lvclass">)  [unwired: 8 in]
            }
          }
          n115 = Scan From String(input string=w283, default 1=Instrument_Types--enum."DAQ" ("Type")) -> (output 1=w286:T6)  [unwired: 3 in, 3 out]
          n116 = call "Cast Instrument to Instrument Type.vi"("error in (no error)"=w289, "Type"=w286, "Instrument in"=w290, "Instrument Classes"=w292) -> ("error out"=w288:errorcluster, "Instrument Classes out"=w291:T9)  [unwired: 5 in, 1 out]
        }
        n117 = Bundle By Name(cluster=w275, "Instruments"=w268) -> (w276:T10)
        n118 = Merge Errors(w273, w267) -> (w274:errorcluster)
        n119 = call <vilib>:"Add State(s) to Queue__jki_lib_state_machine.vi"("State(s) in (\"\")"=w278) -> ("States Out"=w277:string)  [unwired: 14 in]
      }
      frame "Data: Calculate R and G" {
        # "Do not put any code in this frame.\n(It is a separator no-op. You can make a copy of this frame to create a new Data frame)"
        n120 = Unbundle By Name(w311) -> ("Lockin X"=w314:dbl[], "Excitation"=w313:dbl[], "C.E."=w319:refnum<class "Control Experiment.lvclass">)
        n121 = call "Get Channel Indices.vi"("error in (no error)"=w317, "Control Experiment in"=w319) -> ("error out"=w318:errorcluster, "Indices"=w325:T13)  [unwired: 7 in, 1 out]
        n122 = Unbundle By Name(w325) -> ("I+"=w321:i32, "I-"=w320:i32, "V1+"=w323:i32, "V1-"=w324:i32)
        n123 = Less Than 0?(x=w320) -> (x < 0?=w322:bool)
        n124 = Select(t=w321, s=w322, f=w320) -> (s? t:f=w316:i32)
        n125 = call "Calculate R and G (Two Terminal).vi"("Vsource"=w321, "Current"=w316, "AO Amp (V)"=w313, "Lockin []"=w314) -> ("G_2T (Siemens)"=w309:dbl, "R_2T (Ohms)"=w310:dbl)  [unwired: 6 in]
        n126 = call "Calculate R and G (Four Terminal).vi"("V-"=w324, "V+"=w323, "Current"=w316, "Lockin[ ]"=w314) -> ("G_4T (Siemens)"=w303:dbl, "R_4T (ohms)"=w308:dbl)  [unwired: 4 in, 2 out]
        n127 = call "Calculate R and G 2.vi"("Electrodes"="Electrodes", "Excitation"=w313, "Data (V or A)"=w314) -> ("G_4T (S)"=w299:dbl[], "R_4T (Ohms)"=w300:dbl[], "G_2T (S)"=w301:dbl[], "R_2T (Ohms)"=w302:dbl[])  [unwired: 5 in]
        n128 = Build Array (concatenate)(w310, w302) -> (w307:dbl[])
        n129 = Build Array (concatenate)(w309, w301) -> (w306:dbl[])
        n130 = Build Array (concatenate)(w308, w300) -> (w305:dbl[])
        n131 = Build Array (concatenate)(w303, w299) -> (w304:dbl[])
        n132 = Bundle By Name(cluster=w311, "R2T"=w307, "G2T"=w306, "R4T"=w305, "G4T"=w304) -> (w312:T10)
        n133 = call <vilib>:"Add State(s) to Queue__jki_lib_state_machine.vi"("State(s) in (\"\")"=w327) -> ("States Out"=w326:string)  [unwired: 14 in]
      }
      frame "Data: Cleanup" {
        # "Cleanup any data and references, here.\n(this is called automatically, by the Macro: Exit)"
        n134 = Unbundle By Name(w345) -> ("Transport"=w346:refnum<class "Transport.lvclass">, "Execution:State"=w342:T11, "C.E."=w340:refnum<class "Control Experiment.lvclass">, "Instruments"=w339:T9, "Core.Current VI Reference"=w333:refnum<vi>)
        n135 = case shown="\"Run top level\"" w342 {
          tunnel: [w351 w356] -> w338
          tunnel: w340 -> [w351 w355]
          tunnel: w341 -> [w350 w353]
          tunnel: [w350 w354] -> w336
          tunnel: w339 -> [w349 w352]
          tunnel: [w349 w352] -> w334
          frame Default {
          }
          frame "Run top level" {
            n136 = call "Close Dictionary.vi"("error in (no error)"=w353, "Control Experiment in"=w355) -> ("error out"=w354:errorcluster, "Control Experiment out"=w356:refnum<class "Control Experiment.lvclass">)  [unwired: 8 in]
          }
        }
        n137 = call "Write Instruments.vi"("error in (no error)"=w336, "Instruments"=w334, "Control Experiment in"=w338) -> ("error out"=w335:errorcluster, "Control Experiment out"=w337:refnum<class "Control Experiment.lvclass">)  [unwired: 7 in]
        n138 = call "Write Dependencies.vi"("error in (no error)"=w335, "Control Experiment"=w337, "Transport in"=w346) -> ("error out"=w329:errorcluster, "Transport out"=w331:refnum<class "Transport.lvclass">)  [unwired: 7 in]
        n139 = call "Send RunningStatus Notifier.vi"("error in (no error)"=w329, "Running?"=FALSE, "Transport in"=w331) -> ("error out"=w328:errorcluster, "Transport out"=w330:refnum<class "Transport.lvclass">)  [unwired: 7 in]
        n140 = Bundle By Name(cluster=w345, "Transport"=w330) -> (w344:T10)
        n141 = Close Reference(reference=w333, error in (no error)=w328) -> (error out=w343:errorcluster)
        n142 = call <vilib>:"Add State(s) to Queue__jki_lib_state_machine.vi"("State(s) in (\"\")"=w348) -> ("States Out"=w347:string)  [unwired: 14 in]
      }
      frame "---------- UI ----------" {
        # "Do not put any code in this frame.\n(It is a separator no-op. You can make a copy of this frame to create a new UI frame)"
        n143 = call <vilib>:"Add State(s) to Queue__jki_lib_state_machine.vi"("State(s) in (\"\")"=w360) -> ("States Out"=w359:string)  [unwired: 14 in]
      }
      frame "UI: Initialize" {
        # "Initialize the User Interface, here.\n(this is called automatically, by the Macro: Init)"
        n144 = invoke on="Stop" class="Bool" method="Reinit To Default"() -> ()  [unwired: 3 in, 3 out]
        n145 = call <userlib>:"Fit VI window to Largest Dec__ogtk.vi"("error in (no error)"=w364, "border spacing (2 px)"=0) -> ("error out"=w362:errorcluster)  [unwired: 4 in, 1 out]
        n146 = call <vilib>:"Add State(s) to Queue__jki_lib_state_machine.vi"("State(s) in (\"\")"=w366) -> ("States Out"=w365:string)  [unwired: 14 in]
      }
      frame "UI: Update Legend (Time Graphs)" {
        n147 = Unbundle By Name(w375) -> ("Lockin X"=w373:dbl[])
        n148 = control-ref of="X"() -> (w371:refnum<vi>)
        n149 = control-ref of="Y"() -> (w370:refnum<vi>)
        n150 = control-ref of="X (2)"() -> (w369:refnum<vi>)
        n151 = control-ref of="Mean"() -> (w368:refnum<vi>)
        n152 = Array Size(array=w373) -> (size(s)=w372:i32)
        n153 = Build Array(w371, w370, w369, w368) -> (w367:refnum<vi>[])
        n154 = for {
          tunnel: w372 -> [w380]
          tunnel: w367 -> [w379] mode=indexing
          tunnel: w376 -> [w382]
          tunnel: [w381] -> w374
          n155 = for {
            N: w380 -> [_]
            tunnel: [w390] -> w381
            tunnel: w382 -> [w389]
            tunnel: w380 -> [w384]
            tunnel: w379 -> [w383]
            i -> [w388]
            n156 = Increment(x=w388) -> (x+1=w387:i32)
            n157 = Format Into String(format string="Lockin %d", w387) -> (resulting string=w386:string)  [unwired: 2 in, 1 out]
            n158 = property on="Property Node" class="XYGraph (strict)"(reference=w383, error in=w389, "Active Plot"=w388, "Plot.Plot Name"=w386, "LegPlotMin"=w384) -> (error out=w385:errorcluster)  [unwired: 1 out]
            n159 = call <vilib>:"Clear Errors.vi"("error in (no error)"=w385) -> ("error out"=w390:errorcluster)  [unwired: 5 in, 1 out]
          }
        }
        n160 = call <vilib>:"Add State(s) to Queue__jki_lib_state_machine.vi"("State(s) in (\"\")"=w378) -> ("States Out"=w377:string)  [unwired: 14 in]
      }
      frame "UI: Update Legend (R G Graphs)" {
        # "R2T (CE)\nR4T (CE)\nR2T (1)\nR4T (1)"
        n161 = control-ref of="R vs time"() -> (w409:refnum<vi>)
        n162 = control-ref of="R vs T"() -> (w403:refnum<vi>)
        n163 = control-ref of="R vs B"() -> (w402:refnum<vi>)
        n164 = control-ref of="G vs time"() -> (w401:refnum<vi>)
        n165 = local read "Electrodes"() -> (w395:T2)
        n166 = Array Size(array=w395) -> (size(s)=w407:i32)
        n167 = Increment(x=w407) -> (x+1=w394:i32)
        n168 = Multiply(x=w394, y=2) -> (x*y=w393:i32)
        n169 = Decrement(x=w393) -> (x-1=w406:i32)
        n170 = Build Array(w409, w403, w402, w401) -> (w408:refnum<vi>[])
        n171 = for {
          N: w406 -> [_]
          tunnel: [w416] -> w399 mode=indexing
          i -> [w417]
          n172 = Increment(x=w417) -> (x+1=w414:i32)
          n173 = Format Into String(format string="%d", w414) -> (resulting string=w416:string)  [unwired: 2 in, 1 out]
        }
        n174 = Build Array (concatenate)("CE" ("format string"), w399) -> (w397:string[])
        n175 = Interleave 1D Arrays(w397, w397) -> (w398:string[])
        n176 = for {
          tunnel: w393 -> [w418]
          tunnel: w408 -> [w422] mode=indexing
          tunnel: w411 -> [w423]
          tunnel: string[] ["R", "R", "R", "G"] -> [w421] mode=indexing
          tunnel: [w419] -> _
          tunnel: [w420] -> w404
          tunnel: w398 -> [w419]
          n177 = for {
            N: w418 -> [_]
            tunnel: w423 -> [w439]
            tunnel: w418 -> [w427]
            tunnel: w422 -> [w438]
            tunnel: w421 -> [w437]
            tunnel: [w435] -> w420
            tunnel: w419 -> [w430] mode=indexing
            i -> [w436]
            n178 = call <userlib>:"MGI True if Odd.vi"("Integer"=w436) -> ("Odd?"=w434:bool)
            n179 = Select(t="4" ("format string"), s=w434, f="2" ("format string")) -> (s? t:f=w433:string)
            n180 = Format Into String(format string="%s%sT (%s)", w437, w433, w430) -> (resulting string=w429:string)  [unwired: 2 in, 1 out]
            n181 = In Range and Coerce(upper limit=6, x=w427, lower limit=2) -> (coerced(x)=w424:i32)  [unwired: 1 out]
            n182 = property on="Property Node" class="XYGraph (strict)"(reference=w438, error in=w439, "Active Plot"=w436, "Plot.Plot Name"=w429, "LegPlotMin"=u32 2 ("Legend:Plot Minimum"), "LegNumRows"=w424) -> (error out=w435:errorcluster)  [unwired: 1 out]
          }
        }
        n183 = call <vilib>:"Clear Errors.vi"("error in (no error)"=w404) -> ("error out"=w405:errorcluster)  [unwired: 5 in, 1 out]
        n184 = call <vilib>:"Add State(s) to Queue__jki_lib_state_machine.vi"("State(s) in (\"\")"=w413) -> ("States Out"=w412:string)  [unwired: 14 in]
      }
      frame "UI: Update Scale Labels" {
        # "Do not put any code in this frame.\n(It is a separator no-op. You can make a copy of this frame to create a new UI frame)"
        n185 = case shown="\"h/e2 & e2/h\"" "Units" {
          tunnel: ["R (ohms)" "R (h/e2)"] -> w443
          tunnel: ["G (siemens)" "G (e2/h)"] -> w441
          frame "ohms & siemens", Default {
          }
          frame "h/e2 & e2/h" {
          }
        }
        n186 = property on="R vs time" class="XYGraph (strict)"("YScale.NameLbl.Text"=w443) -> ()  [unwired: 2 in, 2 out]
        n187 = property on="G vs time" class="XYGraph (strict)"("YScale.NameLbl.Text"=w441) -> ()  [unwired: 2 in, 2 out]
        n188 = call <vilib>:"Add State(s) to Queue__jki_lib_state_machine.vi"("State(s) in (\"\")"=w447) -> ("States Out"=w446:string)  [unwired: 14 in]
      }
      frame "UI: Update Status" {
        # "Do not put any code in this frame.\n(It is a separator no-op. You can make a copy of this frame to create a new UI frame)"
        n189 = local read "Instrument Status"() -> (w456:string)
        n190 = To Lower Case(string=w452) -> (all lower case string=w461:string)
        n191 = Equal?(x=w461, y="reset") -> (x = y?=w460:bool)
        n192 = Empty String/Path?(string/path=w456) -> (empty?=w455:bool)
        n193 = Format Into String(format string="%s, %s", w456, w452) -> (resulting string=w454:string)  [unwired: 2 in, 1 out]
        n194 = Select(t=w452, s=w455, f=w454) -> (s? t:f=w453:string)
        n195 = Select(t="", s=w460, f=w453) -> (s? t:f=→"Instrument Status":string)
        n196 = call <vilib>:"Add State(s) to Queue__jki_lib_state_machine.vi"("State(s) in (\"\")"=w466) -> ("States Out"=w465:string)  [unwired: 14 in]
      }
      frame "UI: Cursor Set" {
        # "Argument"
        # "Set and Unset Cursor Busy.\n(Usage: \"UI: Cursor Set >> Busy|Idle\")"
        n197 = case shown="\"Idle\", Default" w467 {
          tunnel: w469 -> [w474 w476]
          tunnel: [w473 w475] -> w468
          frame "Idle", Default {
            n198 = call <vilib>:"Unset Busy.vi"("error in (no error)"=w474) -> ("error out"=w473:errorcluster)  [unwired: 10 in]
          }
          frame "Busy" {
            n199 = call <vilib>:"Set Busy.vi"("error in (no error)"=w476) -> ("error out"=w475:errorcluster)  [unwired: 9 in, 1 out]
          }
        }
        n200 = call <vilib>:"Add State(s) to Queue__jki_lib_state_machine.vi"("State(s) in (\"\")"=w472) -> ("States Out"=w471:string)  [unwired: 14 in]
      }
      frame "UI: Front Panel State" {
        # "Argument"
        # "Set Front Panel Open or Closed\n(Usage: \"UI: Front Panel State >> Open|Close\")"
        n201 = Unbundle By Name(w479) -> ("Core.Current VI Reference"=w478:refnum<vi>)
        n202 = case shown="\"Open\", \"Standard\", Default" w477 {
          tunnel: w481 -> [w489 w504 w515 w528 w541]
          tunnel: [w491 w505 w517 w530 w543] -> w480
          tunnel: w478 -> [w490 w502 w516 w529 w542]
          frame "Open", "Standard", Default {
            w484 = T4."Standard" ("State")
            n203 = property class="VI"(reference=w490, error in=w489) -> (reference out=w487:refnum<vi>, error out=w488:errorcluster, "FP.State"=w486:T4)
            n204 = Not Equal?(x=w486, y=w484) -> (x != y?=w485:bool)
            n205 = case shown="False" w485 {
              tunnel: [w495 w497] -> w491
              tunnel: w488 -> [w494 w497]
              tunnel: w487 -> [w493 _]
              tunnel: w484 -> [w492 _]
              frame True {
                n206 = invoke class="VI" method="FP.Open"(reference=w493, error in=w494, "Activate"=TRUE, "State"=w492) -> (error out=w495:errorcluster)  [unwired: 1 in, 4 out]
              }
              frame False {
              }
            }
          }
          frame "Close", "Closed" {
            n207 = property class="VI"(reference=w502, error in=w504) -> (reference out=w501:refnum<vi>, error out=w503:errorcluster, "FP.State"=w499:T4)
            n208 = Not Equal?(x=w499, y=T4."Closed" ("Front Panel Window:State")) -> (x != y?=w498:bool)
            n209 = case shown="True" w498 {
              tunnel: [w506 w509] -> w505
              tunnel: w503 -> [w506 w508]
              tunnel: w501 -> [_ w507]
              frame False {
              }
              frame True {
                n210 = invoke class="VI" method="FP.Close"(reference=w507, error in=w508) -> (error out=w509:errorcluster)  [unwired: 1 in, 2 out]
              }
            }
          }
          frame "Hidden", "Hide" {
            w510 = T4."Hidden" ("State")
            n211 = property class="VI"(reference=w516, error in=w515) -> (reference out=w513:refnum<vi>, error out=w514:errorcluster, "FP.State"=w512:T4)
            n212 = Not Equal?(x=w512, y=w510) -> (x != y?=w511:bool)
            n213 = case shown="True" w511 {
              tunnel: [w521 w522] -> w517
              tunnel: w514 -> [w520 w522]
              tunnel: w513 -> [w519 _]
              tunnel: w510 -> [w518 _]
              frame True {
                n214 = invoke class="VI" method="FP.Open"(reference=w519, error in=w520, "State"=w518) -> (error out=w521:errorcluster)  [unwired: 2 in, 4 out]
              }
              frame False {
              }
            }
          }
          frame "Minimize", "Minimized" {
            w523 = T4."Minimized" ("State")
            n215 = property class="VI"(reference=w529, error in=w528) -> (reference out=w526:refnum<vi>, error out=w527:errorcluster, "FP.State"=w525:T4)
            n216 = Not Equal?(x=w525, y=w523) -> (x != y?=w524:bool)
            n217 = case shown="True" w524 {
              tunnel: [w534 w535] -> w530
              tunnel: w527 -> [w533 w535]
              tunnel: w526 -> [w532 _]
              tunnel: w523 -> [w531 _]
              frame True {
                n218 = invoke class="VI" method="FP.Open"(reference=w532, error in=w533, "State"=w531) -> (error out=w534:errorcluster)  [unwired: 2 in, 4 out]
              }
              frame False {
              }
            }
          }
          frame "Maximize", "Maximized" {
            w536 = T4."Maximized" ("State")
            n219 = property class="VI"(reference=w542, error in=w541) -> (reference out=w539:refnum<vi>, error out=w540:errorcluster, "FP.State"=w538:T4)
            n220 = Not Equal?(x=w538, y=w536) -> (x != y?=w537:bool)
            n221 = case shown="True" w537 {
              tunnel: [w547 w548] -> w543
              tunnel: w540 -> [w546 w548]
              tunnel: w539 -> [w545 _]
              tunnel: w536 -> [w544 _]
              frame True {
                n222 = invoke class="VI" method="FP.Open"(reference=w545, error in=w546, "State"=w544) -> (error out=w547:errorcluster)  [unwired: 2 in, 4 out]
              }
              frame False {
              }
            }
          }
        }
        n223 = call <vilib>:"Add State(s) to Queue__jki_lib_state_machine.vi"("State(s) in (\"\")"=w483) -> ("States Out"=w482:string)  [unwired: 14 in]
      }
      frame "UI: Update Graphs" {
        # "YUK"
        n224 = Unbundle By Name(w593) -> ("time"=w558:dbl, "R2T"=w566:dbl[], "R4T"=w560:dbl[], "G2T"=w561:dbl[], "G4T"=w562:dbl[], "temperature"=w591:dbl, "magnet field"=w592:dbl, "angle"=w557:dbl)
        n225 = To Lower Case(string=w596) -> (all lower case string=w594:string)
        n226 = Equal?(x=w594, y="reset") -> (x = y?=w559:bool)
        n227 = local read "Units"() -> (w582:enum16{"ohms & siemens", "h/e2 & e2/h"})
        n228 = Build Array(w591) -> (w563:dbl[])
        n229 = Build Array(w592) -> (w564:dbl[])
        n230 = Build Array(w557) -> (w556:dbl[])
        n231 = case shown="\"ohms & siemens\", Default" w582 {
          tunnel: [1.0 ("Siemens/(e2/h)") w613] -> w583
          frame "ohms & siemens", Default {
          }
          frame "h/e2 & e2/h" {
            w613 = 3.874046e-05  # Siemens/(e2/h)
          }
        }
        n232 = call "Graph Lockin vs Parameter.vi"("reset?"=w559, "Y"=w556, "X"=w558) -> ("Data vs Parameter"=w555:cluster{dbl[], dbl[]}[])  [unwired: 8 in]
        n233 = call "Graph Lockin vs Parameter.vi"("reset?"=w559, "Y"=w566, "X"=w558) -> ("Data vs Parameter"=w565:cluster{dbl[], dbl[]}[])  [unwired: 8 in]
        n234 = call "Graph Lockin vs Parameter.vi"("reset?"=w559, "Y"=w560, "X"=w558) -> ("Data vs Parameter"=w585:cluster{dbl[], dbl[]}[])  [unwired: 8 in]
        n235 = call "Graph Lockin vs Parameter.vi"("reset?"=w559, "Y"=w561, "X"=w558) -> ("Data vs Parameter"=w590:cluster{dbl[], dbl[]}[])  [unwired: 8 in]
        n236 = call "Graph Lockin vs Parameter.vi"("reset?"=w559, "Y"=w562, "X"=w558) -> ("Data vs Parameter"=w588:cluster{dbl[], dbl[]}[])  [unwired: 8 in]
        n237 = call "Graph Lockin vs Parameter.vi"("reset?"=w559, "Y"=w563, "X"=w558) -> ("Data vs Parameter"=w578:cluster{dbl[], dbl[]}[])  [unwired: 8 in]
        n238 = call "Graph Lockin vs Parameter.vi"("reset?"=w559, "Y"=w564, "X"=w558) -> ("Data vs Parameter"=w577:cluster{dbl[], dbl[]}[])  [unwired: 8 in]
        n239 = Index Array(array=w555) -> (element=w554:cluster{dbl[], dbl[]})  [unwired: 1 in]
        n240 = call-poly <vilib>:"Multiply.vi"("y (1)"=w583, "XY-data"=w565) -> ("XY-data out"=w586:cluster{"X-array":dbl[], "Y-array":dbl[]}[])  [unwired: 8 in, 1 out]
        n241 = call-poly <vilib>:"Multiply.vi"("y (1)"=w583, "XY-data"=w585) -> ("XY-data out"=w584:cluster{"X-array":dbl[], "Y-array":dbl[]}[])  [unwired: 8 in, 1 out]
        n242 = call-poly <vilib>:"Divide.vi"("y (1)"=w583, "XY-data"=w590) -> ("XY-data out"=w589:cluster{"X-array":dbl[], "Y-array":dbl[]}[])  [unwired: 8 in, 1 out]
        n243 = call-poly <vilib>:"Divide.vi"("y (1)"=w583, "XY-data"=w588) -> ("XY-data out"=w587:cluster{"X-array":dbl[], "Y-array":dbl[]}[])  [unwired: 8 in, 1 out]
        n244 = Index Array(array=w578) -> (element=w572:cluster{dbl[], dbl[]})  [unwired: 1 in]
        n245 = Index Array(array=w577) -> (element=w573:cluster{dbl[], dbl[]})  [unwired: 1 in]
        n246 = call-poly <vilib>:"Get X and Y.vi"("XY-data"=w554) -> ("Y-array"=w551:dbl[], "XY-data out"=w549:cluster{"X-array":dbl[], "Y-array":dbl[]})  [unwired: 7 in, 2 out]
        n247 = Build Array(w549) -> (→"Angle vs time":cluster{"X-array":dbl[], "Y-array":dbl[]}[])
        n248 = Interleave 1D Arrays(w586, w584) -> (w581:cluster{"X-array":dbl[], "Y-array":dbl[]}[])
        n249 = Interleave 1D Arrays(w589, w587) -> (→"G vs time":cluster{"X-array":dbl[], "Y-array":dbl[]}[])
        n250 = call-poly <vilib>:"Get X and Y.vi"("XY-data"=w581) -> ("Y-Arrays"=w552:cluster{"Y-array":dbl[]}[], "XY-data out"=→"R vs time":cluster{"X-array":dbl[], "Y-array":dbl[]}[])  [unwired: 7 in, 2 out]
        n251 = call-poly <vilib>:"Get X and Y.vi"("XY-data"=w572) -> ("Y-array"=w567:dbl[], "XY-data out"=w576:cluster{"X-array":dbl[], "Y-array":dbl[]})  [unwired: 7 in, 2 out]
        n252 = call-poly <vilib>:"Get X and Y.vi"("XY-data"=w573) -> ("Y-array"=w574:dbl[], "XY-data out"=w575:cluster{"X-array":dbl[], "Y-array":dbl[]})  [unwired: 7 in, 2 out]
        n253 = for {
          tunnel: w567 -> [w605]
          tunnel: w552 -> [w607] mode=indexing
          tunnel: [w604] -> w568 mode=indexing
          n254 = Unbundle(w607) -> ("Y-array"=w606:dbl[])
          n255 = call <vilib>:"Initialize.vi"("Y-array"=w606, "X-array"=w605) -> ("XY-data out"=w604:cluster{"X-array":dbl[], "Y-array":dbl[]})  [unwired: 8 in, 1 out]
        }
        "R vs T" <- w568
        n256 = for {
          tunnel: w574 -> [w609]
          tunnel: w552 -> [w611] mode=indexing
          tunnel: [w608] -> w571 mode=indexing
          n257 = Unbundle(w611) -> ("Y-array"=w610:dbl[])
          n258 = call <vilib>:"Initialize.vi"("Y-array"=w610, "X-array"=w609) -> ("XY-data out"=w608:cluster{"X-array":dbl[], "Y-array":dbl[]})  [unwired: 8 in, 1 out]
        }
        "R vs B" <- w571
        n259 = for {
          tunnel: w551 -> [w601]
          tunnel: w552 -> [w603] mode=indexing
          tunnel: [w600] -> w553 mode=indexing
          n260 = Unbundle(w603) -> ("Y-array"=w602:dbl[])
          n261 = call <vilib>:"Initialize.vi"("Y-array"=w602, "X-array"=w601) -> ("XY-data out"=w600:cluster{"X-array":dbl[], "Y-array":dbl[]})  [unwired: 8 in, 1 out]
        }
        "R vs Angle" <- w553
        n262 = Build Array(w576) -> (→"T vs time":cluster{"X-array":dbl[], "Y-array":dbl[]}[])
        n263 = Build Array(w575) -> (→"B vs time":cluster{"X-array":dbl[], "Y-array":dbl[]}[])
        n264 = call <vilib>:"Add State(s) to Queue__jki_lib_state_machine.vi"("State(s) in (\"\")"=w599) -> ("States Out"=w598:string)  [unwired: 14 in]
      }
      frame "UI: Update Lockin Graphs" {
        n265 = Unbundle By Name(w627) -> ("time"=w620:dbl, "Lockin X"=w619:dbl[], "time"=w618:dbl, "Lockin Y"=w617:dbl[], "time"=w616:dbl, "Lockin Mean"=w615:dbl[])
        n266 = To Lower Case(string=w624) -> (all lower case string=w625:string)
        n267 = Equal?(x=w625, y="reset") -> (x = y?=w614:bool)
        n268 = call "Graph Lockin vs Parameter.vi"("reset?"=w614, "Y"=w619, "X"=w620) -> ("Data vs Parameter"=→"X" →"X (2)":cluster{dbl[], dbl[]}[])  [unwired: 8 in]
        n269 = call "Graph Lockin vs Parameter.vi"("reset?"=w614, "Y"=w617, "X"=w618) -> ("Data vs Parameter"=→"Y":cluster{dbl[], dbl[]}[])  [unwired: 8 in]
        n270 = call "Graph Lockin vs Parameter.vi"("reset?"=w614, "Y"=w615, "X"=w616) -> ("Data vs Parameter"=→"Mean":cluster{dbl[], dbl[]}[])  [unwired: 8 in]
        n271 = call <vilib>:"Add State(s) to Queue__jki_lib_state_machine.vi"("State(s) in (\"\")"=w630) -> ("States Out"=w629:string)  [unwired: 14 in]
      }
      frame "---------- Macro ----------" {
        # "Do not put any code in this frame.\n(It is a separator no-op. You can make a copy of this frame to create a new Macro frame)"
        n272 = call <vilib>:"Add State(s) to Queue__jki_lib_state_machine.vi"("State(s) in (\"\")"=w634) -> ("States Out"=w633:string)  [unwired: 14 in]
      }
      frame "Macro: Initialize" {
        # "Initialization Macro\n(This is called once, when the VI starts)"
        n273 = call <vilib>:"Add State(s) to Queue__jki_lib_state_machine.vi"("State(s) in Front (\"\")"="Data: Initialize\nInitialize Core Data\nUI: Initialize\nUI: Front Panel State >> Open\nData: Initialize Top Level\n\nMacro: Initialize Instruments\nMacro: Measure\n\nUI: Update Legend (Time Graphs)\nUI: Update Legend (R G Graphs)\nUI: Update Scale Labels\nUI: Update Lockin Graphs >> reset\nUI: Update Graphs >> reset\n// File: Save >> reset\nFile: Write JSON", "State(s) in (\"\")"=w639) -> ("States Out"=w638:string)  [unwired: 13 in]
      }
      frame "Macro: Measure" {
        # "Initialization Macro\n(This is called once, when the VI starts)"
        n274 = call <vilib>:"Add State(s) to Queue__jki_lib_state_machine.vi"("State(s) in Front (\"\")"="UI: Update Status >> reset\nMeasure: Time\nMacro: Measure Instruments\nData: Calculate R and G\nUI: Update Lockin Graphs\nUI: Update Graphs\nFile: Save\nData: Check Notifier\nIdle //Service Event Structure", "State(s) in (\"\")"=w644) -> ("States Out"=w643:string)  [unwired: 13 in]
      }
      frame "Macro: Initialize Instruments" {
        # "Do not put any code in this frame.\n(It is a separator no-op. You can make a copy of this frame to create a new Macro frame)"
        n275 = call <vilib>:"Add State(s) to Queue__jki_lib_state_machine.vi"("State(s) in Front (\"\")"="Data: Initialize Instruments\nData: Disable Unsupported Instruments\nData: Open Instruments\nData: Configure Magnet Type" ("State(s) in Front (\"\")"), "State(s) in (\"\")"=w649) -> ("States Out"=w648:string)  [unwired: 13 in]
      }
      frame "Macro: Measure Instruments" {
        # "Do not put any code in this frame.\n(It is a separator no-op. You can make a copy of this frame to create a new Macro frame)"
        n276 = Unbundle By Name(w657) -> ("Instruments"=w655:T9)
        n277 = Cluster To Array(cluster=w655) -> (array=w654:refnum<class "Instrument.lvclass">[])
        n278 = for {
          tunnel: w654 -> [w665] mode=indexing
          tunnel: [w668] -> w650 mode=indexing if=w663
          tunnel: [w661] -> w653 mode=indexing
          n279 = call "Get IsConfigured.vi"("SMO"=w665) -> ("error out"=w662:errorcluster, "IsConfigured?"=w663:bool, "SMO out"=w664:refnum<class "Instrument.lvclass">)  [unwired: 8 in]
          n280 = call "Get StateName.vi"("error in (no error)"=w662, "SMO"=w664) -> ("error out"=w661:errorcluster, "StateName"=w666:string)  [unwired: 7 in, 1 out]
          n281 = Concatenate Strings("Measure: " ("string"), w666) -> (w668:string)
        }
        n282 = Merge Errors(w651, w653) -> (w652:errorcluster)
        n283 = call <vilib>:"1D String Array to Delimited String.vi"("delimiter"="\n", "string array"=w650) -> ("delimited string"=w656:string)  [unwired: 9 in]
        n284 = call <vilib>:"Add State(s) to Queue__jki_lib_state_machine.vi"("State(s) in Front (\"\")"=w656, "State(s) in (\"\")"=w660) -> ("States Out"=w659:string)  [unwired: 13 in]
      }
      frame "Macro: Magnet Hold" {
        # "Do not put any code in this frame.\n(It is a separator no-op. You can make a copy of this frame to create a new Macro frame)"
        n285 = call <vilib>:"Add State(s) to Queue__jki_lib_state_machine.vi"("State(s) in Front (\"\")"="Idle //Service Event Structure\nUI: Update Status >> reset\nMeasure: Temperature", "State(s) in (\"\")"=w673) -> ("States Out"=w672:string)  [unwired: 13 in]
      }
      frame "Macro: Exit" {
        # "Exit Macro\n(This is called once, when the VI exits)"
        n286 = Unbundle By Name(w681) -> ("Core.Close Panel on Exit?"=w680:bool)
        n287 = Select(t="UI: Front Panel State >> Close", s=w680, f="") -> (s? t:f=w677:string)
        n288 = call <vilib>:"Add State(s) to Queue__jki_lib_state_machine.vi"("State(s) in Front (\"\")"="Data: Close Instruments", "State(s) in (\"\")"=w677, "State(s) at Back (\"\")"="Data: Cleanup\nExit") -> ("States Out"=w675:string)  [unwired: 12 in]
        n289 = call <vilib>:"Add State(s) to Queue__jki_lib_state_machine.vi"("State(s) in Front (\"\")"=w675, "State(s) in (\"\")"=w684) -> ("States Out"=w683:string)  [unwired: 13 in]
      }
      frame "---------- File ----------" {
        # "Template Separator\n(You can make a copy of, or modify, this frame)"
        n290 = call <vilib>:"Add State(s) to Queue__jki_lib_state_machine.vi"("State(s) in (\"\")"=w688) -> ("States Out"=w687:string)  [unwired: 14 in]
      }
      frame "File: Save" {
        # "Your code here.\n(You can make a copy of, or modify, this frame)"
        n291 = Unbundle By Name(w708) -> ("C.E."=w698:refnum<class "Control Experiment.lvclass">, "AO"=w705:dbl[], "AI"=w704:dbl[], "Lockin X"=w703:dbl[], "Lockin Y"=w702:dbl[])
        n292 = To Lower Case(string=w690) -> (all lower case string=w691:string)
        n293 = Not Equal?(x=w691, y="reset") -> (x != y?=w689:bool)
        n294 = Build Cluster Array(w705, w704, w703, w702) -> (w701:cluster{"Lockin Y":dbl[]}[])
        n295 = for {
          shift-right: [w715] -> w696
          shift-left: w693 -> [w711]
          tunnel: string[] ["AO", "AI", "X", "Y"] -> [w712] mode=indexing
          tunnel: [w714] -> w697 mode=concatenating
          tunnel: w701 -> [w713] mode=indexing
          n296 = call "Data to Dictionary.vim"("Error in"=w711, "Data in"=w713, "Label in"=w712) -> ("Error out"=w715:errorcluster, "Data out"=w714:T14[])  [unwired: 7 in]
        }
        n297 = call "Write Dictionary Elements (Loop).vi"("error in (no error)"=w696, "Data in"=w697, "Control Experiment in"=w698) -> ("error out"=w695:errorcluster, "Control Experiment out"=w699:refnum<class "Control Experiment.lvclass">)  [unwired: 7 in]
        n298 = call "Save Transport TDMS File.vi"("append?"=w689, "error in (no error)"=w695, "Control Experiment in"=w699) -> ("error out"=w694:errorcluster, "Control Experiment out"=w700:refnum<class "Control Experiment.lvclass">)  [unwired: 7 in]
        n299 = Bundle By Name(cluster=w708, "C.E."=w700) -> (w707:T10)
        n300 = call <vilib>:"Add State(s) to Queue__jki_lib_state_machine.vi"("State(s) in (\"\")"=w710) -> ("States Out"=w709:string)  [unwired: 14 in]
      }
      frame "File: Write JSON" {
        # "Template Separator\n(You can make a copy of, or modify, this frame)"
        n301 = Unbundle By Name(w716) -> ("C.E."=w722:refnum<class "Control Experiment.lvclass">)
        n302 = call "Write JSON to Dictionary.vi"("error in (no error)"=w720, "Control Experiment in"=w722) -> ("error out"=w719:errorcluster, "Control Experiment out"=w721:refnum<class "Control Experiment.lvclass">)  [unwired: 8 in]
        n303 = disable-structure shown="Disabled" {
          disable-tunnel: [w730 w734] -> w723
          disable-tunnel: w721 -> [w729 w734]
          disable-tunnel: w719 -> [w728 w733]
          disable-tunnel: [w727 w733] -> w718
          frame Disabled {
            w726 = cluster{"test":string, "refresh (ms)":u32} {"test"="some text", "refresh (ms)"=1000}  # test cluster
            n304 = call "To JSON Text.vim"("error in (no error)"=w728, "Anything"=w726) -> ("error out"=w727:errorcluster, "<JSON>"=w732:string)  [unwired: 8 in]
            n305 = call "Write Dictionary Element.vi"("value"=w732, "key"="<LockinTime>", "Control Experiment in"=w729) -> ("Control Experiment out"=w730:refnum<class "Control Experiment.lvclass">)  [unwired: 7 in, 1 out]
          }
          frame Enabled {
          }
        }
        n306 = Bundle By Name(cluster=w716, "C.E."=w723) -> (w717:T10)
        n307 = call <vilib>:"Add State(s) to Queue__jki_lib_state_machine.vi"("State(s) in (\"\")"=w725) -> ("States Out"=w724:string)  [unwired: 14 in]
      }
      frame "---------- Measure ----------" {
        # "Do not put any code in this frame.\n(It is a separator no-op. You can make a copy of this frame to create a new Macro frame)"
        n308 = call <vilib>:"Add State(s) to Queue__jki_lib_state_machine.vi"("State(s) in (\"\")"=w738) -> ("States Out"=w737:string)  [unwired: 14 in]
      }
      frame "Measure: Time" {
        # "Measure: Time.\n()"
        n309 = Unbundle By Name(w742) -> ("C.E."=w745:refnum<class "Control Experiment.lvclass">)
        n310 = Get Date/Time In Seconds() -> (seconds since 1Jan1904=w747:timestamp)
        n311 = To Double Precision Float(number=w747) -> (double precision float=w743:dbl)
        n312 = call "Write Dictionary Element.vi"("error in (no error)"=w739, "value"=w743, "key"="Time", "Control Experiment in"=w745) -> ("error out"=w740:errorcluster, "Control Experiment out"=w746:refnum<class "Control Experiment.lvclass">)  [unwired: 6 in]
        n313 = Bundle By Name(cluster=w742, "C.E."=w746, "time"=w743) -> (w741:T10)
        n314 = call <vilib>:"Add State(s) to Queue__jki_lib_state_machine.vi"("State(s) in (\"\")"=w749) -> ("States Out"=w748:string)  [unwired: 14 in]
      }
      frame "Measure: Temperature" {
        # "Measure: Temperature.\n(called dynamically if instrument is configured in Control Experiment.vi)"
        n315 = Unbundle By Name(w762) -> ("Instruments.Temperature"=w763:refnum<class "Instrument.Cryostat.lvclass">, "C.E."=w766:refnum<class "Control Experiment.lvclass">)
        n316 = call-dynamic "getTemperature.vi"("error in (no error)"=w760, "Instrument.Cryostat in"=w763) -> ("error out"=w759:errorcluster, "Temperature (K)"=w750:dbl, "Instrument.Cryostat out"=w765:refnum<class "Instrument.Cryostat.lvclass">)  [unwired: 5 in, 2 out]
        n317 = Greater Or Equal?(x=w750, y="T_hold (K)") -> (x >= y?=w753:bool)
        n318 = And(x=w753, y="Hold?") -> (x .and. y?=w754:bool)
        n319 = call "Write Dictionary Element.vi"("error in (no error)"=w759, "value"=w750, "key"="Temperature", "Control Experiment in"=w766) -> ("error out"=w757:errorcluster, "Control Experiment out"=w764:refnum<class "Control Experiment.lvclass">)  [unwired: 6 in]
        n320 = case shown="No Error" w757 {
          selector: w757 -> [w781 w786]
          tunnel: w750 -> [w784 _]
          tunnel: [w779 _] -> w758
          tunnel: [w781 w786] -> w756
          tunnel: w754 -> [w777 _]
          frame No Error {
            n321 = call <userlib>:"Boolean Trigger__ogtk.vi"("Boolean Input"=w777) -> ("Rising Edge"=w774:bool, "Falling Edge"=w769:bool)  [unwired: 1 in]
            n322 = Format Into String(format string="T = %2f K", w784) -> (resulting string=w782:string)  [unwired: 2 in, 1 out]
            n323 = Select(t="Macro: Magnet Hold" ("format string"), s=w774, f="") -> (s? t:f=w775:string)
            n324 = Select(t="Macro: Magnet UnHold", s=w769, f="") -> (s? t:f=w771:string)
            n325 = call <vilib>:"Build State String with Arguments__JKI_lib_State_Machine.vi"("Arguments (\"\")"=w782, "State"="UI: Update Status" ("format string")) -> ("State with Arguments"=w778:string)  [unwired: 4 in]
            n326 = Select(t=w775, s=w777, f=w771) -> (s? t:f=w780:string)
            n327 = call <vilib>:"Add State(s) to Queue__jki_lib_state_machine.vi"("State(s) in Front (\"\")"=w778, "State(s) at Back (\"\")"=w780) -> ("States Out"=w779:string)  [unwired: 13 in]
          }
          frame Error {
          }
        }
        n328 = Bundle By Name(cluster=w762, "Instruments.Temperature"=w765, "C.E."=w764, "temperature"=w750) -> (w761:T10)
        n329 = call <vilib>:"Add State(s) to Queue__jki_lib_state_machine.vi"("State(s) in Front (\"\")"=w758, "State(s) in (\"\")"=w768) -> ("States Out"=w767:string)  [unwired: 13 in]
      }
      frame "Measure: Magnet" {
        # "Measure: Magnet.\n(called dynamically by if instrument is configured in Control Experiment.vi)"
        n330 = Unbundle By Name(w795) -> ("Instruments.Magnet"=w797:refnum<class "Instrument.Cryostat.lvclass">, "C.E."=w800:refnum<class "Control Experiment.lvclass">)
        n331 = call-dynamic "getMagnet.vi"("error in (no error)"=w793, "Instrument.Cryostat in"=w797) -> ("error out"=w792:errorcluster, "B Field (T)"=w788:dbl, "Instrument.Cryostat out"=w799:refnum<class "Instrument.Cryostat.lvclass">)  [unwired: 5 in, 2 out]
        n332 = call "Calculate dBdt.vi"("B Field (T)"=w788) -> ("dB/dt (T/min)"=w787:dbl)  [unwired: 10 in]
        n333 = call "Write Dictionary Element.vi"("error in (no error)"=w792, "value"=w788, "key"="Magnet", "Control Experiment in"=w800) -> ("error out"=w791:errorcluster, "Control Experiment out"=w798:refnum<class "Control Experiment.lvclass">)  [unwired: 6 in]
        n334 = case shown="No Error" w791 {
          selector: w791 -> [w810 w815]
          tunnel: w788 -> [w813 _]
          tunnel: [w810 w815] -> w790
          tunnel: w787 -> [w806 _]
          tunnel: [w803 _] -> w789
          frame No Error {
            n335 = Format Into String(format string="B = %2f T", w813) -> (resulting string=w811:string)  [unwired: 2 in, 1 out]
            n336 = Format Into String(format string="dB/dt = %2f T/min", w806) -> (resulting string=w809:string)  [unwired: 2 in, 1 out]
            n337 = call <vilib>:"Build State String with Arguments__JKI_lib_State_Machine.vi"("Arguments (\"\")"=w811, "State"="UI: Update Status" ("format string")) -> ("State with Arguments"=w805:string)  [unwired: 4 in]
            n338 = call <vilib>:"Build State String with Arguments__JKI_lib_State_Machine.vi"("Arguments (\"\")"=w809, "State"="UI: Update Status" ("format string")) -> ("State with Arguments"=w804:string)  [unwired: 4 in]
            n339 = call <vilib>:"Add State(s) to Queue__jki_lib_state_machine.vi"("State(s) in Front (\"\")"=w805, "State(s) at Back (\"\")"=w804) -> ("States Out"=w803:string)  [unwired: 13 in]
          }
          frame Error {
          }
        }
        n340 = Bundle By Name(cluster=w795, "Instruments.Magnet"=w799, "C.E."=w798, "magnet field"=w788, "magnet rate"=w787) -> (w794:T10)
        n341 = call <vilib>:"Add State(s) to Queue__jki_lib_state_machine.vi"("State(s) in Front (\"\")"=w789, "State(s) in (\"\")"=w802) -> ("States Out"=w801:string)  [unwired: 13 in]
      }
      frame "Measure: Hold Magnet" {
        # "Measure: Hold Magnet.\n(It is a separator no-op. You can make a copy of this frame to create a new Macro frame)"
        n342 = Unbundle By Name(w831) -> ("magnet rate"=w816:dbl, "Instruments.Magnet"=w821:refnum<class "Instrument.Cryostat.lvclass">)
        n343 = call-dynamic "getMagnetTarget.vi"("error in (no error)"=w819, "Instrument.Cryostat in"=w821) -> ("error out"=w820:errorcluster, "B Field (T)"=w817:dbl, "Instrument.Cryostat out"=w818:refnum<class "Instrument.Cryostat.lvclass">)  [unwired: 5 in, 2 out]
        n344 = call-dynamic "getMagnet.vi"("error in (no error)"=w820, "Instrument.Cryostat in"=w818) -> ("error out"=w824:errorcluster, "B Field (T)"=w829:dbl, "Instrument.Cryostat out"=w827:refnum<class "Instrument.Cryostat.lvclass">)  [unwired: 5 in, 2 out]
        n345 = call-dynamic "setMagnet.vi"("Mode"=Magnet_Mode--Enum."Driven", "error in (no error)"=w824, "Target Rate (T/min)"=0.1, "Target Field (T)"=w829, "Instrument.Cryostat in"=w827) -> ("error out"=w823:errorcluster, "Instrument.Cryostat out"=w826:refnum<class "Instrument.Cryostat.lvclass">)  [unwired: 5 in]
        n346 = Bundle By Name(cluster=w831, "magnet rate hold"=w816, "magnet hold"=w817, "Instruments.Magnet"=w826) -> (w830:T10)
        n347 = call <vilib>:"Add State(s) to Queue__jki_lib_state_machine.vi"("State(s) in Front (\"\")"="" ("State(s) in Front (\"\")"), "State(s) in (\"\")"=w833) -> ("States Out"=w832:string)  [unwired: 13 in]
      }
      frame "Measure: UnHold Magnet" {
        # "Measure: Hold Magnet.\n(It is a separator no-op. You can make a copy of this frame to create a new Macro frame)"
        n348 = Unbundle By Name(w843) -> ("Instruments.Magnet"=w837:refnum<class "Instrument.Cryostat.lvclass">, "magnet hold"=w834:dbl, "magnet rate hold"=w835:dbl)
        n349 = call-dynamic "setMagnet.vi"("Mode"=Magnet_Mode--Enum."Driven", "error in (no error)"=w836, "Target Rate (T/min)"=w835, "Target Field (T)"=w834, "Instrument.Cryostat in"=w837) -> ("error out"=w839:errorcluster, "Instrument.Cryostat out"=w841:refnum<class "Instrument.Cryostat.lvclass">)  [unwired: 5 in]
        n350 = Bundle By Name(cluster=w843, "Instruments.Magnet"=w841) -> (w842:T10)
        n351 = call <vilib>:"Add State(s) to Queue__jki_lib_state_machine.vi"("State(s) in Front (\"\")"="" ("State(s) in Front (\"\")"), "State(s) in (\"\")"=w845) -> ("States Out"=w844:string)  [unwired: 13 in]
      }
      frame "Measure: Vector Magnet" {
        # "Measure: Vector Magnet.\n(called dynamically by if instrument is configured in Control Experiment.vi)"
        n352 = Unbundle By Name(w864) -> ("Instruments.Magnet"=w853:refnum<class "Instrument.Cryostat.lvclass">, "C.E."=w848:refnum<class "Control Experiment.lvclass">)
        n353 = case shown="\"X\"" "Axis" {
          tunnel: [2 ("index") 0 ("index") 1 ("index")] -> w856
          frame "Z", Default {
          }
          frame "X" {
          }
          frame "Y" {
          }
        }
        n354 = call-dynamic "getMagnetVector.vi"("error in (no error)"=w852, "Instrument.Cryostat in"=w853) -> ("error out"=w850:errorcluster, "Field (T)"=w846:dbl[], "Instrument.Cryostat out"=w855:refnum<class "Instrument.Cryostat.lvclass">)  [unwired: 5 in, 2 out]
        n355 = for {
          tunnel: string[] ["Bx", "By", "Bz"] ("input 1") -> [w870] mode=indexing
          tunnel: w846 -> [w869] mode=indexing
          shift-right: [w871] -> w847
          shift-left: w848 -> [w872]
          tunnel: w850 -> [w868]
          tunnel: [w867] -> w849
          n356 = call "Write Dictionary Element.vi"("error in (no error)"=w868, "value"=w869, "key"=w870, "Control Experiment in"=w872) -> ("error out"=w867:errorcluster, "Control Experiment out"=w871:refnum<class "Control Experiment.lvclass">)  [unwired: 6 in]
        }
        n357 = Index Array(array=w846, index #4=w856) -> (element #1=w861:dbl, element #2=w860:dbl, element #3=w859:dbl, element #4=w854:dbl)  [unwired: 3 in]
        n358 = case shown="No Error" w849 {
          selector: w849 -> [w878 w884]
          tunnel: w861 -> [w882 _]
          tunnel: [w879 _] -> w858
          tunnel: [w878 w884] -> w862
          tunnel: w860 -> [w877 _]
          tunnel: w859 -> [w876 _]
          frame No Error {
            n359 = Format Into String(format string="B = [%2f, %2f, %2f]", w882, w877, w876) -> (resulting string=w880:string)  [unwired: 2 in, 1 out]
            n360 = call <vilib>:"Build State String with Arguments__JKI_lib_State_Machine.vi"("Arguments (\"\")"=w880, "State"="UI: Update Status" ("format string")) -> ("State with Arguments"=w879:string)  [unwired: 4 in]
          }
          frame Error {
          }
        }
        n361 = Bundle By Name(cluster=w864, "Instruments.Magnet"=w855, "C.E."=w847, "magnet field"=w854) -> (w863:T10)
        n362 = call <vilib>:"Add State(s) to Queue__jki_lib_state_machine.vi"("State(s) in Front (\"\")"=w858, "State(s) in (\"\")"=w866) -> ("States Out"=w865:string)  [unwired: 13 in]
      }
      frame "Measure: Capacitance" {
        # "Measure: Capacitance.\n(called dynamically if instrument is configured in Control Experiment.vi)"
        n363 = Unbundle By Name(w889) -> ("Instruments.Capacitance"=w895:refnum<class "Instrument.CBridge.lvclass">, "C.E."=w896:refnum<class "Control Experiment.lvclass">)
        n364 = call-dynamic "getCapacitance.vi"("error in (no error)"=w891, "Instrument.CBridge in"=w895) -> ("error out"=w892:errorcluster, "Capacitance (pF)"=w886:dbl, "Instrument.CBridge out"=w894:refnum<class "Instrument.CBridge.lvclass">)  [unwired: 7 in]
        n365 = call "Write Dictionary Element.vi"("error in (no error)"=w892, "value"=w886, "key"="Capacitance", "Control Experiment in"=w896) -> ("error out"=w888:errorcluster, "Control Experiment out"=w897:refnum<class "Control Experiment.lvclass">)  [unwired: 6 in]
        n366 = case shown="No Error" w888 {
          selector: w888 -> [w900 w906]
          tunnel: w886 -> [w904 _]
          tunnel: [w901 _] -> w885
          tunnel: [w900 w906] -> w887
          frame No Error {
            n367 = Format Into String(format string="C = %2f pF", w904) -> (resulting string=w902:string)  [unwired: 2 in, 1 out]
            n368 = call <vilib>:"Build State String with Arguments__JKI_lib_State_Machine.vi"("Arguments (\"\")"=w902, "State"="UI: Update Status" ("format string")) -> ("State with Arguments"=w901:string)  [unwired: 4 in]
          }
          frame Error {
          }
        }
        n369 = Bundle By Name(cluster=w889, "Instruments.Capacitance"=w894, "C.E."=w897) -> (w890:T10)
        n370 = call <vilib>:"Add State(s) to Queue__jki_lib_state_machine.vi"("State(s) in Front (\"\")"=w885, "State(s) in (\"\")"=w899) -> ("States Out"=w898:string)  [unwired: 13 in]
      }
      frame "Measure: Strain Cell" {
        # "Measure: Strain Cell.\n(called dynamically if instrument is configured in Control Experiment.vi)"
        n371 = Unbundle By Name(w911) -> ("Instruments.Strain Cell"=w917:refnum<class "Instrument.Strain.lvclass">, "C.E."=w918:refnum<class "Control Experiment.lvclass">)
        n372 = call-dynamic "getStrain.vi"("error in (no error)"=w913, "Instrument.Strain in"=w917) -> ("error out"=w914:errorcluster, "Strain (V)"=w908:dbl, "Instrument.Strain out"=w916:refnum<class "Instrument.Strain.lvclass">)  [unwired: 7 in]
        n373 = call "Write Dictionary Element.vi"("error in (no error)"=w914, "value"=w908, "key"="Strain", "Control Experiment in"=w918) -> ("error out"=w910:errorcluster, "Control Experiment out"=w919:refnum<class "Control Experiment.lvclass">)  [unwired: 6 in]
        n374 = case shown="No Error" w910 {
          selector: w910 -> [w922 w928]
          tunnel: w908 -> [w926 _]
          tunnel: [w923 _] -> w907
          tunnel: [w922 w928] -> w909
          frame No Error {
            n375 = Format Into String(format string="Strain = %2f V", w926) -> (resulting string=w924:string)  [unwired: 2 in, 1 out]
            n376 = call <vilib>:"Build State String with Arguments__JKI_lib_State_Machine.vi"("Arguments (\"\")"=w924, "State"="UI: Update Status" ("format string")) -> ("State with Arguments"=w923:string)  [unwired: 4 in]
          }
          frame Error {
          }
        }
        n377 = Bundle By Name(cluster=w911, "Instruments.Strain Cell"=w916, "C.E."=w919) -> (w912:T10)
        n378 = call <vilib>:"Add State(s) to Queue__jki_lib_state_machine.vi"("State(s) in Front (\"\")"=w907, "State(s) in (\"\")"=w921) -> ("States Out"=w920:string)  [unwired: 13 in]
      }
      frame "Measure: Delay Line" {
        # "Measure: Delay Line.\n(called dynamically if instrument is configured in Control Experiment.vi)"
        n379 = Unbundle By Name(w933) -> ("Instruments.Delay Line"=w939:refnum<class "Instrument.DelayLine.lvclass">, "C.E."=w940:refnum<class "Control Experiment.lvclass">)
        n380 = call-dynamic "getDelay.vi"("error in (no error)"=w935, "Instrument.DelayLine in"=w939) -> ("error out"=w936:errorcluster, "delay (ps)"=w930:dbl, "Instrument.DelayLine out"=w938:refnum<class "Instrument.DelayLine.lvclass">)  [unwired: 6 in, 1 out]
        n381 = call "Write Dictionary Element.vi"("error in (no error)"=w936, "value"=w930, "key"="Delay", "Control Experiment in"=w940) -> ("error out"=w932:errorcluster, "Control Experiment out"=w941:refnum<class "Control Experiment.lvclass">)  [unwired: 6 in]
        n382 = case shown="No Error" w932 {
          selector: w932 -> [w944 w950]
          tunnel: w930 -> [w948 _]
          tunnel: [w945 _] -> w929
          tunnel: [w944 w950] -> w931
          frame No Error {
            n383 = Format Into String(format string="Delay = %2f ps", w948) -> (resulting string=w946:string)  [unwired: 2 in, 1 out]
            n384 = call <vilib>:"Build State String with Arguments__JKI_lib_State_Machine.vi"("Arguments (\"\")"=w946, "State"="UI: Update Status" ("format string")) -> ("State with Arguments"=w945:string)  [unwired: 4 in]
          }
          frame Error {
          }
        }
        n385 = Bundle By Name(cluster=w933, "Instruments.Delay Line"=w938, "C.E."=w941) -> (w934:T10)
        n386 = call <vilib>:"Add State(s) to Queue__jki_lib_state_machine.vi"("State(s) in Front (\"\")"=w929, "State(s) in (\"\")"=w943) -> ("States Out"=w942:string)  [unwired: 13 in]
      }
      frame "Measure: Rotator" {
        # "Measure: Rotator.\n(called dynamically if instrument is configured in Control Experiment.vi)"
        n387 = Unbundle By Name(w955) -> ("Instruments.Rotator"=w961:refnum<class "Instrument.Cryostat.lvclass">, "C.E."=w962:refnum<class "Control Experiment.lvclass">)
        n388 = call-dynamic "getAngle.vi"("error in (no error)"=w957, "Instrument.Cryostat in"=w961) -> ("error out"=w958:errorcluster, "Angle (°)"=w951:dbl, "Instrument.Cryostat out"=w960:refnum<class "Instrument.Cryostat.lvclass">)  [unwired: 5 in, 2 out]
        n389 = call "Write Dictionary Element.vi"("error in (no error)"=w958, "value"=w951, "key"="Angle", "Control Experiment in"=w962) -> ("error out"=w954:errorcluster, "Control Experiment out"=w963:refnum<class "Control Experiment.lvclass">)  [unwired: 6 in]
        n390 = case shown="No Error" w954 {
          selector: w954 -> [w966 w972]
          tunnel: w951 -> [w970 _]
          tunnel: [w967 _] -> w952
          tunnel: [w966 w972] -> w953
          frame No Error {
            n391 = Format Into String(format string="Angle = %2f°", w970) -> (resulting string=w968:string)  [unwired: 2 in, 1 out]
            n392 = call <vilib>:"Build State String with Arguments__JKI_lib_State_Machine.vi"("Arguments (\"\")"=w968, "State"="UI: Update Status" ("format string")) -> ("State with Arguments"=w967:string)  [unwired: 4 in]
          }
          frame Error {
          }
        }
        n393 = Bundle By Name(cluster=w955, "Instruments.Rotator"=w960, "C.E."=w963, "angle"=w951) -> (w956:T10)
        n394 = call <vilib>:"Add State(s) to Queue__jki_lib_state_machine.vi"("State(s) in Front (\"\")"=w952, "State(s) in (\"\")"=w965) -> ("States Out"=w964:string)  [unwired: 13 in]
      }
      frame "Measure: DAQ" {
        # "Do not put any code in this frame.\n(It is a separator no-op. You can make a copy of this frame to create a new Macro frame)"
        n395 = Unbundle By Name(w996) -> ("Instruments.DAQ"=w976:refnum<class "Instrument.LockinAPI.lvclass">)
        n396 = call "Cast Lockin tsc.vi"("error in (no error)"=w973, "Instrument.LockinAPI in"=w976) -> ("error out"=w974:errorcluster, "Instrument.Lockin out"=w975:refnum<class "Instrument.Lockin.lvclass">)  [unwired: 8 in]
        n397 = call-dynamic "getAOconfig.vi"("error in (no error)"=w974, "Instrument.Lockin in"=w975) -> ("error out"=w987:errorcluster, "AOconfig"=w990:T15, "Instrument.Lockin out"=w989:refnum<class "Instrument.Lockin.lvclass">)  [unwired: 7 in]
        n398 = call-dynamic "getResults.vi"("error in (no error)"=w987, "Instrument.Lockin in"=w989) -> ("error out"=w979:errorcluster, "Results (Dictionary)"=w991:cluster{"key":string, "value":dbl}[], "Instrument.Lockin out"=w988:refnum<class "Instrument.Lockin.lvclass">)  [unwired: 6 in, 1 out]
        n399 = call <userlib>:"Parse Results (all).vi"("Type"=Results_Type--Enum."X", "error in (no error)"=w979, "Results (Dictionary)"=w991) -> ("error out"=w994:errorcluster, "Data"=w986:dbl[], "Results (Dictionary)"=w995:cluster{"key":string, "value":dbl}[])  [unwired: 5 in, 1 out]
        "X Channels" <- w986
        n400 = call <userlib>:"Parse Results (all).vi"("Type"=Results_Type--Enum."Y", "error in (no error)"=w994, "Results (Dictionary)"=w995) -> ("error out"=w983:errorcluster, "Data"=w985:dbl[], "Results (Dictionary)"=w984:cluster{"key":string, "value":dbl}[])  [unwired: 5 in, 1 out]
        "Y Channels" <- w985
        n401 = call <userlib>:"Parse Results (all).vi"("Type"=Results_Type--Enum."Mean", "error in (no error)"=w983, "Results (Dictionary)"=w984) -> ("error out"=w980:errorcluster, "Data"=w977:dbl[])  [unwired: 5 in, 2 out]
        "Mean" <- w977
        n402 = for {
          tunnel: [w1002] -> w981 mode=indexing
          tunnel: w990 -> [w1001] mode=indexing
          tunnel: [w1000] -> w978 mode=indexing
          n403 = Unbundle By Name(w1001) -> ("Amplitude"=w1002:dbl, "Offset"=w1000:dbl)
        }
        n404 = Bundle By Name(cluster=w996, "Instruments.DAQ"=w988, "Lockin X"=w986, "Lockin Y"=w985, "Lockin Mean"=w977, "Excitation"=w981, "AO"=w978, "AI"=w977) -> (w997:T10)
        n405 = call <vilib>:"Add State(s) to Queue__jki_lib_state_machine.vi"("State(s) in (\"\")"=w999) -> ("States Out"=w998:string)  [unwired: 14 in]
      }
      frame "Measure: DAQ Waveforms" {
        n406 = Unbundle By Name(w1006) -> ("Instruments.DAQ"=w1005:refnum<class "Instrument.LockinAPI.lvclass">)
        n407 = disable-structure shown="Enabled" {
          disable-tunnel: [w1023 w1031] -> w1007
          disable-tunnel: w1006 -> [w1022 w1031]
          disable-tunnel: w1005 -> [w1012 _]
          disable-tunnel: [w1016 w1030] -> w1004
          disable-tunnel: w1003 -> [w1011 w1030]
          frame Disabled {
            n408 = call "Cast Lockin tsc.vi"("error in (no error)"=w1011, "Instrument.LockinAPI in"=w1012) -> ("error out"=w1010:errorcluster, "Instrument.Lockin out"=w1013:refnum<class "Instrument.Lockin.lvclass">)  [unwired: 8 in]
            n409 = call-dynamic "getAIwfm.vi"("error in (no error)"=w1010, "Instrument.Lockin in"=w1013) -> ("error out"=w1018:errorcluster, "AI Waveform"=w1015:waveform(dbl)[], "Instrument.Lockin out"=w1019:refnum<class "Instrument.Lockin.lvclass">)  [unwired: 7 in]
            n410 = call-dynamic "getAOwfm.vi"("error in (no error)"=w1018, "Instrument.Lockin in"=w1019) -> ("error out"=w1016:errorcluster, "AO Waveforrm"=w1020:waveform(dbl)[], "Instrument.Lockin out"=w1017:refnum<class "Instrument.Lockin.lvclass">)  [unwired: 7 in]
            n411 = for {
              tunnel: w1020 -> [w1029] mode=indexing
              tunnel: [w1027] -> w1021 mode=indexing
              n412 = Unbundle By Name(w1029) -> ("Y"=w1028:dbl[])
              n413 = Index Array(array=w1028) -> (element=w1027:dbl)  [unwired: 1 in]
            }
            n414 = for {
              tunnel: w1015 -> [w1026] mode=indexing
              tunnel: [w1024] -> w1014 mode=indexing
              n415 = Unbundle By Name(w1026) -> ("Y"=w1025:dbl[])
              n416 = Index Array(array=w1025) -> (element=w1024:dbl)  [unwired: 1 in]
            }
            n417 = Bundle By Name(cluster=w1022, "Instruments.DAQ"=w1017, "AO"=w1021, "AI"=w1014) -> (w1023:T10)
          }
          frame Enabled {
            # "#154"
          }
        }
        n418 = call <vilib>:"Add State(s) to Queue__jki_lib_state_machine.vi"("State(s) in (\"\")"=w1009) -> ("States Out"=w1008:string)  [unwired: 14 in]
      }
    }
  }
  "error out" <- w3
  n419 = Unbundle By Name(w2) -> ("Transport"=→"Transport out":refnum<class "Transport.lvclass">)
